vi "p2.vi"() -> ()   [LabVIEW 2021, in "d21.lvlib"]
uses:
  d21.lvlib
  <vilib>/regexp/Match Regular Expression.xnode
  AOC/AOC.lvlib
panel:
  out "Numeric":i64
  out "String":string
  out "Reduced 2":string
  out "Reduced 1":string
  out "side 2":string
  out "side 1":string
  in  "Example":bool
  in  "Example":string="root: pppw + sjmn\ndbpl: 5\ncczh: sllz + lgvd\nzczc: 2\nptdq: humn - dvpt\ndvpt: 3\nlfqf: 4\nhumn: 5\nljgn: 2\nsjmn: drzm * dbpl\nsllz: 4\npppw: cczh / lfqf\nlgvd: ljgn * ptdq\ndrzm: hmdt - zczc\nhmdt: 32"
  in  "variables":string[](array[string])=["fqsj", "fdlt", "zgmz", "rhjl", "snpj", "zvhz", "rldg", "lmll", "stps", "jwbt", "fpmq", "ffpf", "mmmv", "gbzb", "cfjs", "cncf", "mfnp", "jhgz", "mgft", "mrrb", "zllz", "zpdc", "fzvp", "mnmv", "hqfj", "dzjs", "grzz", "zmgd", "mrhm", "pgsb", "hlzf", "qnpr", "fnmj", "nsmc", "dbbn", "gtff", "wrbt", "ztsz", "pqcs", "wlst", "ffls", "ljjm", "vftj", "pggh", "wqpn", "mmmm", "gnfc", "cqnp", "sbvb", "vsmc", "humn", "ggrg", "vccs", "mrgq", "gpgw", "sqrl", "mncr", "rtdb", "lpbw", "ggtj", "drbw", "ztfd", "cbzs", "hhrm", "pnwq", "cwml", "cpbh", "gmmv", "wcrw", "mvgg", "jfcq", "jjpz", "rlqj", "zpgv", "crjg", "bvdp", "hplw", "tfzv", "fnhp", "hzrr", "jstf", "nblh", "lhfc", "wppw", "bdlj", "rpwp", "fbqb", "csrw", "vvwv", "czsz", "pmpb", "fwhb", "bthq", "mzzm", "jngd", "zjqs", "hsbt", "bqtv", "wztp", "hvhf", "fzbh", "bjmt", "bdps", "psqs", "jfpt", "cnpc", "pwdp", "vvmw", "jvzp", "jzsb", "smcz", "hvng", "lftw", "wtvv", "bbbr", "sqsh", "hwbl", "fpnh", "pbrm", "chfb", "zjgv", "rcjj", "whlc", "sgnd", "fhgn", "hzmf", "fztw", "fhpw", "ljvp", "jlqf", "lltd", "vlqj", "tzsm", "mrfb", "ftfr", "lqzb", "pfds", "bbzg", "qgpm", "nlvd", "hgvp", "cnpz", "glsj", "tsrp", "rcdp", "qzml", "mvjr", "gvbp", "dcps", "qjdp", "mqbr", "llbh", "llnq", "zlrl", "ngnd", "vfqn", "grdz", "wtwh", "vhhr", "vtpt", "zjzt", "fdzj", "pgjn", "cbmt", "hpvg", "mmvc", "vhsv", "ffzt", "tcmz", "gctb", "pmrt", "hrvj", "sffd", "mlzs", "qjhc", "qbts", "wpts", "nzlb", "ndpz", "rgqg", "vpdz", "pwbs", "rglt", "dqvg", "pssq", "qvst", "hcjh", "jmzp", "wsnt", "rwgw", "ldzg", "rrtc", "wcpv", "bdlb", "bfcs", "bzzp", "mlrt", "mqzz", "fscv", "qnzd", "nscj", "wrfr", "frbf", "ztfh", "qtmg", "lpft", "vjdn", "rbjt", "ppjv", "cddb", "jqlb", "whvm", "zrwj", "vmzb", "lhwg", "czlv", "vhqj", "svjl", "qrdp", "qnnj", "fbft", "rlbm", "lwlr", "rntv", "cmrf", "tpwz", "mwrq", "lmpr", "zgct", "btcg", "qqwq", "qqdg", "hhqs", "tcgz", "hrsv", "sfjc", "ljhp", "fjzg", "qlfw", "qmjl", "dwms", "szzp", "lvwn", "cmps", "svmc", "fdsq", "ctjd", "gcnn", "pfzr", "jwbq", "mvgf", "wvbq", "ptrm", "hfpm", "tjnh", "vfjf", "pfsj", "vrqf", "ghlb", "pftd", "gsmz", "sjsf", "frtl", "pdhz", "mjbv", "lpwh", "ggzf", "rsbl", "jvct", "wwvz", "ftdw", "stgd", "fdbj", "prgn", "rbgc", "bftf", "lclz", "dspc", "pvzz", "wpjr", "whpl", "mphw", "gnmc", "lnwd", "pcnz", "zznq", "jsml", "sncr", "hhfh", "bbdp", "nqjt", "vsqz", "jdnl", "brhj", "jzmd", "ncdn", "vshf", "psbr", "gznp", "wctd", "qtwp", "pdfn", "shlz", "bqjd", "dssj", "gfwp", "sftl", "lghz", "lwvr", "gjtf", "mmgq", "vqgh", "lmfp", "nbrl", "tlvq", "fjlj", "zrsl", "psgj", "rqmm", "lghr", "lsph", "ztvv", "lwdq", "dmwc", "stwl", "tjsv", "bjbq", "phvh", "gwnp", "lrsm", "qvrn", "rrbs", "pmtv", "rqqf", "twvr", "qqsh", "bwhd", "twvm", "ntnd", "qgrq", "fbjg", "cwbp", "fhtd", "vstv", "hnzz", "fhtv", "hlvn", "fjgb", "vngd", "fccw", "wjpw", "jwzf", "jlvd", "cbcq", "zglp", "nwsv", "hvlr", "rdzq", "bvpn", "hgbm", "qrfg", "gdzt", "tmsq", "pvqg", "vtcj", "bvnt", "pqvc", "zmdn", "qhhl", "sflv", "fsrv", "vvfh", "qbrd", "wgtg", "fthz", "lztw", "hgbc", "fnsr", "lzrf", "qrzs", "vrmn", "cnhc", "whmz", "mcwn", "frrm", "scgw", "jtnp", "dwcc", "nczg", "srbq", "phmc", "wblm", "wchj", "pfsf", "ddwc", "zfff", "vszw", "tnqs", "qmjd", "mpln", "ngpw", "nlnr", "dgsm", "lblg", "grqr", "bfhd", "vwvw", "sgdz", "jsjj", "lzwl", "vpzl", "mqqv", "qtdj", "gjjm", "hpqm", "blqg", "jmrg", "jhsf", "nljz", "djqs", "vhrt", "zqhq", "fqff", "fbcg", "qcwg", "flnv", "qngj", "nzss", "bzhf", "nrhf", "gqhp", "qcfb", "ppnj", "dqbc", "qzsc", "vldv", "bhmq", "rdph", "hhpv", "qtpd", "mrnq", "zfcf", "nvpt", "cdtw", "vthn", "gvmw", "drvd", "nzwf", "rzdl", "cmtj", "jzgc", "trmn", "mdjv", "qfnr", "lmrt", "djzb", "jzjm", "stfl", "jwtf", "hwfw", "gpzf", "pzln", "qgjn", "pvms", "twpc", "cnhl", "fsss", "fvjg", "vnhg", "mmpg", "pmcg", "vmhs", "hfdg", "vjvm", "qsdf", "jfnj", "hmpr", "lndp", "fqph", "lddz", "zjvf", "qfsm", "zgbc", "wdbr", "cfwf", "fmvm", "glvv", "zdlb", "vmjp", "swrj", "pnbt", "tflg", "cvbb", "wrsc", "hvwn", "bmvv", "pbmz", "dspb", "njfr", "vngz", "jqwn", "lhbv", "sjvn", "sccd", "fnhn", "thrp", "djjw", "cpss", "thhv", "sdlc", "dwcs", "zmmg", "jhbp", "zpbt", "cptw", "thqn", "cvjd", "qwfl", "swft", "flcm", "vjvq", "wppp", "gscs", "tjqd", "ssqz", "mlpt", "qshb", "lmhg", "vlqw", "vnjt", "qbtz", "psmz", "bldp", "zlvb", "zldr", "jfpc", "jhfb", "dznt", "qjsm", "wfdf", "ntzq", "dtzp", "jmnq", "pdrl", "rrsr", "ndmt", "vzrw", "cpwh", "mpcq", "dllf", "hhrg", "vqpd", "frtz", "lfrj", "jnwf", "mlmw", "shzm", "ghsv", "wvvd", "bjpf", "dzdz", "bgps", "gstb", "zscg", "wspb", "njmt", "ccfn", "ttsg", "flhq", "clgf", "hpml", "gssz", "bwvv", "nrbl", "wrvb", "cqfp", "sjdv", "hqvl", "mmdv", "wdlq", "fqtj", "hqcw", "pzsw", "bbwd", "cmwv", "zsdb", "zpps", "jhrr", "tcgc", "zgts", "mwwh", "jvbp", "htgt", "sjhh", "tzbj", "rshs", "gjlq", "nbht", "dgrp", "mlwr", "brqf", "vtwf", "crzd", "hwfv", "znrs", "wptb", "qvmv", "fqbs", "mbsr", "qddw", "psmg", "gtlz", "fbnh", "czbt", "mrfd", "gmsl", "nsqh", "trhr", "jmvf", "cbcp", "mssw", "vlth", "rppw", "vcbq", "mbln", "zlth", "vnmj", "gmdz", "tcnw", "hrqc", "jzdw", "lhcc", "wlcf", "vppv", "wpfs", "mzbt", "llwp", "lhlt", "gqth", "jgpl", "gfsn", "hdqf", "mrsr", "gffp", "vnlv", "tmcn", "bgdj", "drzl", "gnzj", "rqbt", "sjpv", "cjtd", "rwth", "jrcm", "gcfh", "lfsw", "gwhg", "msjr", "wcsg", "vtjc", "jrrm", "svdj", "wrnn", "zqns", "fgvl", "jtqc", "hhgq", "ntvw", "pqsm", "gpgv", "fdpb", "srdz", "znqr", "qvtc", "pptp", "czcv", "qszg", "lncj", "rmfw", "ssfw", "rlzq", "dzqz", "pllt", "dcbw", "jnzs", "stjp", "lrwf", "whch", "wpfl", "btqv", "dqvh", "fcgl", "czzd", "gjbv", "prdj", "fgsg", "pptj", "svvz", "zvql", "zwzz", "vrpt", "mwhr", "wcth", "jdvt", "ftcc", "gsdv", "zgnh", "gfrp", "dbhf", "trbc", "ctsb", "wdvw", "lfrq", "wgnp", "mgqq", "lcvr", "lcbg", "qbrw", "rctg", "brpp", "lhwf", "gvht", "njsn", "zbfn", "zpmb", "dqwn", "llfn", "grwz", "dslc", "ndms", "jdzb", "pcbr", "swhv", "qvnm", "dmbb", "vjjj", "fmhp", "jmqw", "bpzj", "dtnn", "ssbz", "jwzp", "shqb", "tpbv", "fgbj", "sqjn", "hbwt", "szlm", "wthv", "bgvh", "thpr", "gddt", "nvwg", "hvgn", "cprg", "gssl", "qlhm", "nbmq", "wrmr", "sdbp", "phtq", "dvhs", "hgsq", "zzzq", "lvmh", "ngwp", "bwgh", "sgnf", "lnrv", "jsvl", "zrqs", "fnzf", "rgnn", "jpsn", "lscv", "cmdh", "tnlt", "dwzf", "mbpn", "hvqw", "qfcb", "flpq", "cchp", "mwmj", "bvfh", "jtth", "tccw", "cjdw", "lngs", "vnhq", "lgnr", "cnlq", "qqpg", "rhwd", "dfwl", "jplw", "ljmz", "rlfr", "nlqz", "gqbc", "dwtr", "zdmt", "pbtd", "zcfd", "gljm", "gcqm", "jqwf", "wjvr", "lnnn", "qwgr", "zlnf", "dbqv", "bclj", "srjd", "bjzg", "plzs", "grhj", "gnjd", "twhl", "nnnd", "thhh", "nhhp", "bfzr", "rcgg", "zrff", "rjmj", "fvss", "fzqd", "tlfp", "mnqb", "ghsl", "bwmb", "jmjw", "msrj", "vwfn", "gpss", "vmgm", "ndhs", "ghlg", "zfrc", "zggn", "bhgs", "rfqr", "blzh", "lvfl", "mpqv", "gqbg", "spbp", "mfcr", "mrdg", "msjl", "twqt", "crnq", "gfjb", "fzjs", "nmlg", "zdgg", "vrzn", "bdhr", "trrb", "smmh", "gpmb", "zlwh", "bhsp", "zplf", "wtzd", "hbqg", "tvvw", "wzvf", "jtss", "vwqm", "jvfm", "ljpj", "shjf", "jfhp", "zdrn", "jgqb", "rqvr", "bhlz", "vlsv", "tjhj", "zcbt", "jbmw", "thjq", "fflh", "vdbm", "ngrc", "ftqq", "lwcv", "czlg", "dlpz", "dmjl", "llfl", "gdmq", "qdwp", "ddzl", "pnhs", "bbfv", "wndp", "bprt", "cvnz", "jfhm", "zflq", "nbgq", "shpf", "bjfv", "dslt", "hchb", "nlgj", "lwpl", "rtcr", "qvhb", "qzhv", "tfqj", "vdmh", "ftdt", "jvrr", "hqth", "vblt", "nprq", "msvm", "dslb", "vpmj", "vdgc", "bfzf", "mhww", "wcjm", "nftf", "wjjn", "qmlr", "tbjd", "sppt", "rdpp", "vbln", "tdfr", "hfrg", "nqzc", "tdwc", "ccwq", "nblt", "rtrm", "gfht", "swgf", "wbwr", "jvsf", "fwzl", "sdsh", "lwlw", "vnts", "qnzq", "qsmb", "qdqj", "nszq", "cpsb", "blpc", "dsql", "vvfm", "ldfr", "hgzd", "ztwf", "ftzl", "wdtb", "mpjc", "tmfg", "mbvw", "fvzt", "rjvd", "msmm", "bpvm", "twjg", "gpcz", "wjfv", "pnft", "swtz", "jljb", "rdms", "qcrj", "tmwh", "rfgp", "ggsw", "tvjg", "qpjg", "pbll", "pbpm", "mdtr", "msqs", "jgsd", "btqc", "rqmd", "sgzm", "srpc", "znqt", "wvgg", "sbrh", "tzsq", "fczq", "fhwj", "bdbl", "pgzr", "fjgt", "jfwh", "srnq", "bvbp", "qlrc", "mlbn", "fdnn", "mmql", "wsql", "tpbz", "ddwg", "lllp", "qmhc", "qhhm", "dmlq", "vlfs", "hrqv", "zjhq", "cbvf", "wgmq", "spgf", "hpcs", "rrnb", "jgrj", "vhcd", "vpfm", "tplj", "gchb", "gzsb", "gqdq", "fpbb", "wbgb", "gpml", "lszf", "rnqw", "dbvt", "tqlv", "rvgs", "qcqd", "drjs", "bfsl", "nldh", "wsbf", "fcfh", "tdjm", "pwwg", "ldgg", "bvjj", "tvfq", "jsgm", "sdmq", "vwcg", "bwfb", "rljt", "tqcw", "ncch", "nttz", "cbjm", "zwdd", "smgm", "tffn", "gnnb", "sdbv", "pjmm", "jpgl", "njjh", "bmcl", "mcmt", "rpgd", "mchw", "vnhp", "snnj", "zmwd", "dbdf", "czzm", "gvtc", "pfdf", "qjmt", "jfsl", "ttmw", "zngb", "wdgr", "dzbl", "sdvq", "llhc", "fmhf", "sndl", "rbjh", "jglv", "nrnc", "fvfv", "hsnb", "lpcp", "rlrj", "qpgd", "bwjj", "fmdv", "prqr", "czjq", "rrfg", "lzcr", "mcdq", "qmlb", "lrbz", "rwjl", "cffn", "bsbs", "fszt", "pmsn", "gjcw", "rscq", "vfdv", "jnzd", "mbjv", "rjtp", "bzpv", "vdtv", "bpcz", "qhpn", "fbqq", "snhj", "nrfq", "cwcg", "hdhq", "tvpj", "gmmw", "mszm", "fhrw", "jvth", "lbzw", "mlwq", "dhln", "mrns", "dzmw", "pdbb", "wwbs", "rnwg", "bfvv", "wmnt", "fllv", "vzhn", "djpp", "rhtm", "tbzz", "rwws", "dpfp", "cshg", "svmf", "cztz", "jhps", "zjwz", "rwgf", "qjcv", "zjth", "zzws", "jmtc", "hhds", "qtnh", "dtfm", "mwsq", "cfmq", "rnqc", "zbmq", "drfs", "dwlp", "pzvs", "tvcv", "jzvj", "hnhv", "slch", "dntj", "wmsr", "snpr", "mjcz", "jjsd", "ndjh", "vnqf", "mvnl", "glln", "crsv", "thss", "mczd", "lcnv", "cghq", "brtm", "jqzz", "mqnc", "lcsg", "fbpf", "flmq", "tldr", "qppc", "mqnr", "bhtb", "dsrc", "sgfw", "tdjh", "frgj", "lcrt", "cjpv", "ssmv", "nzbp", "szjl", "htgj", "hpwh", "gvqg", "nmnr", "zfhv", "pzls", "lmqh", "zcgm", "zhpp", "cbsq", "jgwl", "djwz", "vwbh", "nmcz", "wjzt", "slmh", "jpnz", "sscw", "fqgd", "rlsf", "ggqn", "zbgr", "stds", "pptm", "mfjj", "vsps", "pghb", "vhpn", "mbgv", "srjf", "zprj", "hssb", "vflp", "wqmm", "btmf", "lbzn", "crtg", "hvmn", "qpsl", "rphl", "pbrc", "crps", "ftgq", "brcn", "ttqs", "wrqb", "wggj", "prnn", "mfdd", "tfrz", "llgp", "sqfc", "wssw", "vpvh", "tshp", "qwcf", "jthp", "tqzz", "zvlv", "ntcm", "bwgq", "dfsj", "pldw", "nbsw", "prsz", "mhdv", "zddt", "wjwv", "dljs", "nscr", "vnbh", "scsc", "qhsr", "qsmr", "hghr", "sthl", "jmcr", "rtct", "pldc", "sjzp", "fzhh", "wpjq", "bcdz", "ntvp", "vtbv", "bcdf", "tqsj", "ftvr", "wptm", "qzcj", "wtqq", "rmqh", "vhmc", "znhd", "llnm", "swjq", "jfcn", "fwtt", "jbgz", "lttg", "nghw", "shrv", "cwmh", "hvcm", "tsdl", "lpfz", "sppg", "rgjr", "qjrv", "ftgn", "tscj", "ghmp", "cdrs", "gvrj", "vrnt", "rnnm", "hrcn", "rljv", "pngs", "dndl", "wjvv", "lmvc", "vtgj", "jltn", "ssrb", "rlcj", "frth", "zrdd", "lrpl", "lpsz", "dwsf", "lqrd", "qvdw", "smvb", "pzps", "gpvg", "zqms", "hmdj", "bhzh", "cjdg", "nmtj", "szrj", "tnmt", "phhh", "qsqj", "sgtg", "lvvq", "cmct", "qrgf", "lnzb", "bvjn", "mjzr", "zrbt", "jpwq", "smbv", "vdjf", "zmzd", "vnsf", "glmt", "dgmt", "llhz", "spgn", "dwmn", "fmhb", "pzbj", "lrbs", "bpzr", "bnnt", "pjng", "zgwp", "wgvg", "hjvl", "fvrf", "pqml", "nqft", "vmzt", "mrrw", "fzwq", "mnmr", "lcqq", "lpgv", "srgh", "hmpc", "pbtm", "ncvr", "fclv", "zhtg", "vsnh", "lnsc", "tftq", "mzdw", "pgwr", "qzgr", "czmj", "cscn", "lpnp", "zspd", "vdlr", "nzjt", "ndzb", "thsq", "pdhf", "sgzc", "zmrp", "vphg", "lntt", "cbjl", "vqrf", "sscd", "qcbw", "wfgq", "mgrj", "hqnn", "zdzc", "qght", "cfqb", "lwsn", "hfjh", "vbsr", "vlgr", "rqnt", "pqwg", "sldt", "whcp", "lbvn", "nzlz", "gvhg", "mnjc", "qwrl", "mdlt", "ftth", "chdb", "msdt", "pnlt", "rtpj", "ldnm", "fhhg", "zqfz", "mphc", "pqzg", "dhhr", "hpcj", "wmzc", "srnd", "mrzl", "sdqt", "scvs", "wwhm", "sbcq", "wswp", "swrn", "qffm", "pbpn", "rtvw", "wjbj", "hfgl", "msdc", "lrhg", "hvzv", "jpgf", "djwm", "zfwb", "cwlp", "mhrh", "qmgl", "zzbc", "fsmq", "frrt", "zhrq", "lzhh", "lhfq", "dswf", "jjch", "cmqj", "cwff", "bnrb", "ttvg", "mppd", "nrts", "bblj", "cppb", "gqjt", "phfj", "brwz", "gdzm", "hngs", "frdw", "zvlp", "bltn", "vtsm", "rqtc", "sqbv", "tttp", "thfr", "pmbh", "mqhb", "gwcl", "tqzb", "nwvj", "hszf", "gctg", "sfwc", "ntqz", "nsdj", "zzql", "pvcz", "rrzv", "sdvd", "wrpd", "nmqc", "pgss", "vtbm", "ccrg", "vgtv", "dmjb", "jvcw", "svvl", "dphn", "dwjm", "fzcb", "ddtz", "lffw", "qgzh", "dbrp", "glwr", "hntg", "qhqc", "mhqf", "lzjz", "ptnr", "dzwp", "ftbz", "glvf", "gsgq", "vlms", "gnhg", "rzgj", "cvpc", "sbql", "dqrc", "pwjw", "bddl", "qnsd", "bdzz", "qcmn", "fhlm", "mjnm", "wqmw", "sfzr", "wpwz", "ndvz", "hfhh", "gffm", "pvlf", "wcqv", "chnc", "jzvb", "bngc", "ltqm", "rgqw", "gnbz", "wcrt", "qvfd", "ztsf", "dvlf", "trtj", "dttp", "tvmh", "bqgw", "hbtl", "dcqf", "dffz", "mpmp", "jsvs", "srcm", "rbbr", "dgms", "nvbj", "gstr", "nvfs", "lwbg", "vhlb", "rhqq", "hcvj", "qhdp", "mngp", "gtvr", "msjw", "tfvj", "lmss", "zdtw", "dzmt", "zwdt", "cqsm", "fzdn", "gsnn", "sljs", "tvzt", "qhqj", "fpdb", "fngn", "mprs", "ptlc", "pclv", "zgbp", "vjmb", "zqgm", "tqlt", "bltl", "nnbw", "dghd", "rlhg", "bhzd", "dtwn", "zttv", "bvcg", "jvqh", "zqnf", "rrft", "dlrq", "gfwf", "fhqn", "jfdp", "fwzv", "fgrw", "hwfs", "phrb", "vfwv", "hmpw", "wrts", "jnmh", "qljm", "gqss", "rswn", "sgrr", "ttsz", "mhdr", "bqvv", "zlbw", "qqzp", "gbwj", "hfbj", "rlll", "ctdv", "pdsz", "swwq", "tfgv", "djgl", "qgff", "jmmj", "jswr", "fgld", "jnhf", "jwpf", "mslt", "dgrs", "rbbj", "mccm", "njpj", "wgmf", "lplq", "bcqm", "twdm", "vjcp", "cbqz", "zszs", "rwwp", "lddr", "mgnh", "gfws", "zcbr", "cfwq", "jtfr", "gzmz", "vrzv", "drcm", "nrjz", "sbzv", "tvzz", "jcwg", "rhbg", "pmgb", "vpdq", "lpzw", "dnvb", "ncdr", "lfzc", "qzrn", "vtrz", "cpqm", "srcj", "cgqp", "dtnh", "nbrg", "czts", "jzbc", "dvzm", "qtrf", "nhqw", "hpnh", "vdqq", "crpg", "tjhg", "fvtb", "tfcv", "vtdz", "jgbg", "mmrq", "fsgb", "msnr", "rmfl", "rttb", "wcph", "crcm", "zgfq", "stss", "hrcm", "nsld", "bcwq", "spcp", "rnjn", "cfvb", "bjjn", "gbnz", "vbcn", "cwlv", "rvmp", "pggv", "wscv", "mfsv", "qdwz", "vmlt", "snjj", "ccch", "cslz", "chsf", "qqqc", "jjbj", "gcdw", "qqmb", "szdt", "cscc", "ffzw", "wvhd", "wdrq", "sqmn", "wsdb", "cdjp", "dhfw", "vtvq", "rhnn", "gfds", "mjgq", "fvtd", "zwcf", "thzg", "vlzz", "ptht", "nqhb", "vntl", "sbft", "bmdr", "mvzc", "zngw", "zntj", "znhn", "gddc", "nhrw", "qtfm", "cblf", "bwcj", "dhqh", "qbfz", "svsb", "jhhb", "fcpw", "ddpg", "wshd", "srpm", "ntmq", "gjfb", "ccbw", "hgvb", "hccc", "hgmr", "fvbh", "pdbd", "vssp", "fcmb", "mjgp", "mgtb", "plbl", "hmtj", "htwq", "jgjj", "bgsq", "rqmc", "jvfz", "nzfg", "zsdr", "fgzv", "cgzh", "pqdh", "lrzt", "cmgs", "ttnh", "zsvd", "sjpp", "gvph", "lpzh", "tfbw", "dtjl", "ftjr", "gwbc", "zgvs", "hzfg", "lvpc", "pvtr", "twqf", "mcwz", "mntg", "dtcz", "dqrf", "wblw", "bhwd", "smcf", "vgzv", "qmht", "wsqt", "qmwn", "mdql", "jhzs", "zftn", "cpvd", "gsjf", "gnjw", "lvcp", "bswg", "jpjv", "scsp", "jrnp", "sgcs", "qtmp", "bwgm", "bplm", "pntf", "zghm", "fqlj", "fdqg", "bhgp", "prcd", "ggvq", "tdlf", "cgnr", "ncpn", "lnqc", "wmls", "fpgs", "vnpl", "gqqj", "pdtc", "tqlc", "bfwv", "hpvt", "dqvq", "rfmq", "tvnc", "mftf", "vvpv", "pbfn", "rrsp", "chsg", "pmms", "hbcd", "hvsl", "mcwg", "zzmn", "ppdl", "tbrz", "hczv", "fwtv", "qgjt", "vndc", "tmqf", "ljbn", "lnrr", "dgcq", "lzlb", "tcqz", "rrlf", "dzss", "glbg", "dplg", "nbhf", "jdnj", "pcth", "nqzb", "btzd", "htcn", "tmfm", "lvmv", "lzhg", "zzsp", "rcnl", "bmjr", "hjch", "wjsv", "tpcm", "fgfv", "vmhf", "nrnq", "lvwb", "jnnh", "szrq", "glcz", "jwvb", "ffvr", "dmfd", "nhdf", "bsbt", "dfcv", "nvrc", "hmjc", "mhfc", "hbtt", "jbqj", "zvbs", "jjrp", "bmsj", "mvzv", "tvpc", "gnmd", "srcb", "mwnz", "vjgm", "phwh", "vcdc", "qfsh", "sddl", "grdd", "gdjz", "wqsf", "hgmf", "jmfg", "fdhf", "vgbg", "njwh", "tfpd", "rvzd", "rqqv", "glfc", "fzsj", "lbhs", "bvwz", "svzt", "szhv", "lcvv", "htlz", "fvcs", "rwqr", "msbw", "btmn", "hrqf", "zwpw", "rzgm", "gccl", "ndrd", "swfn", "hjbn", "pjnj", "grws", "mnmn", "mgcj", "scmf", "vsbj", "hnzb", "fdrl", "nmhv", "vdgm", "fzrd", "zhvn", "jpfd", "tvms", "pwdd", "jrbd", "pbht", "ftmm", "cqwl", "tntn", "gtpz", "jqwp", "qfcd", "hfrh", "cftd", "gdzr", "tlsn", "ztfv", "jzhc", "pqlj", "chvn", "npvt", "sddq", "tgsj", "dthz", "tbzf", "vmvd", "qqnc", "wfhj", "vsbc", "dlhh", "grjb", "pjnz", "jcnb", "tvqf", "snbl", "mnhw", "jjsb", "ldrc", "zgnn", "frdh", "pcrq", "rzfv", "pslz", "ltrz", "nljm", "njzd", "pnmp", "czph", "tbpp", "wstn", "dztm", "htcp", "fvsr", "rcln", "njmp", "hfzj", "sgcj", "wrrg", "npdp", "npwg", "pdqh", "jzpn", "wrns", "cjnf", "spgg", "mpqd", "rrvr", "npnc", "crjw", "pgdm", "jpgj", "tpjb", "wptr", "whqn", "llsm", "lwsl", "qtdm", "tfjn", "cczs", "tflv", "jzzt", "ptmq", "hlhj", "pzmc", "rnsc", "gfvb", "tsmw", "tnzf", "vhtm", "bjzj", "rnmz", "vjvl", "hlbl", "trnr", "bttd", "tltr", "tvqz", "blqb", "hczq", "vnml", "tdgw", "wjsw", "prwp", "ppms", "nnvv", "gntm", "tdmc", "gczr", "wbcp", "wzjh", "zhgs", "mpvl", "cgjw", "wsnz", "nhgs", "wzmw", "drfl", "dvgl", "gbrl", "cfpd", "gfjg", "rhfj", "fwjz", "gdgp", "ddqh", "zlnt", "fcvj", "fqpd", "wfrm", "dzqs", "pfps", "jbbv", "jqbd", "pzmm", "jfvl", "mrjc", "pbnl", "wvnm", "mzsr", "htwv", "tsjh", "zdwh", "dnrs", "tnvv", "hfqm", "mgfn", "wlql", "mpmb", "jchf", "nnpf", "nqbm", "srwt", "lwjr", "fwpb", "htzl", "cmjq", "gpsl", "bpms", "mnld", "tfhf", "hdjm", "dngs", "hnnt", "mpqq", "hcbs", "rsrp", "wdjp", "mcgr", "clhs", "zppc", "rgfr", "tmqm", "rcdg", "thfg", "bvqd", "rtqw", "lpdr", "wbwh", "gfjq", "bzdv", "bmrn", "njld", "zjct", "tjgg", "rqht", "jlvb", "pfrc", "psdt", "mpfp", "vlhn", "srjh", "tpch", "tthg", "htmn", "shnl", "pffp", "wbzh", "vjst", "jmdw", "hgqg", "njnh", "ctgb", "fmcp", "rwlt", "wjdf", "mhwj", "bqjr", "pvdd", "vdsp", "bmrv", "mjbr", "wnzb", "rthh", "pdmh", "bhzg", "rflc", "jfrl", "bzsj", "fsjh", "swtj", "zlcq", "fjbs", "rbcm", "cmtg", "zhhh", "rjtr", "fbhc", "bdcr", "mphf", "lbfr", "frlj", "rtwl", "qffw", "pbzz", "lgcs", "hbbw", "bffq", "zwch", "jwpq", "fpnb", "ssdl", "jsfw", "lstd", "mgvw", "vzzc", "glmz", "lrfp", "dgvm", "mqcv", "zbsg", "lzqg", "rtrt", "zvdb", "jgtr", "pbbd", "hjcz", "qhfh", "rvwn", "jtgb", "zshv", "twrj", "qqcd", "rwtd", "dffp", "wqts", "nfgf", "vjjm", "stvh", "mvbm", "rzfm", "ztpv", "prbd", "bnqg", "lfct", "zpdt", "fmfs", "mnfn", "lngc", "ntlc", "rnnc", "rrnj", "mnvt", "rlbq", "gsfw", "zfcl", "cmtw", "fjmv", "lccn", "djft", "mrhg", "fjwp", "zzcr", "qgwj", "bjbj", "sngh", "vrlw", "mzfj", "jzzs", "rhjv", "jhnn", "tpbb", "rjln", "bppv", "jtdz", "hvwz", "lnvl", "gbdb", "sjfl", "fwcs", "mrvp", "zpmt", "wbrj", "wrzn", "cgfp", "pdjq", "cqqr", "lgpm", "cphl", "frms", "sdph", "tqwj", "drgt", "jwjf", "bbcz", "wqnz", "vzlj", "dzhv", "sqmd", "mjbs", "wptl", "mctl", "mwlm", "ghrb", "fnhf", "rfss", "zltc", "bfjw", "swfm", "tzhz", "rhqt", "bqbl", "lqtf", "lhtw", "bscl", "stph", "mlbw", "lgvv", "crcs", "ghnz", "qlzb", "mplm", "rlqr", "cpjm", "rvfq", "bcvw", "jlpl", "pbmf", "bcrh", "vbqc", "fmml", "rrhd", "nsrb", "wznm", "zfdg", "tcvs", "jzpm", "bmnh", "mcnq", "trfm", "mtvl", "llfv", "zdjp", "mmqt", "wpcp", "dsfj", "vcgg", "mbvc", "qtlz", "rwcm", "pzrv", "vgwt", "wzsm", "cjmv", "qbwm", "gsrw", "lbvf", "smwp", "zfdm", "mvdl", "wggs", "qwrb", "qrjj", "gdjw", "vvqb", "wltf", "bjhb", "sjsc", "dsvv", "dnsc", "tjwz", "tptw", "dgzb", "jlwv", "bhbz", "fwhn", "drwv", "rtth", "qbvs", "qmws", "vptz", "wlvv", "qjmb", "qzfc", "gdqd", "jbtg", "blrb", "jzsf", "ltsj", "ctwr", "gnrm", "stlg", "fjrb", "dvjz", "gtss", "wlms", "gnhf", "vlnw", "qqhr", "sjsv", "npsg", "hctf", "pdwf", "hplg", "scbr", "lgpf", "prlb", "ppfb", "gmfl", "bmhv", "nvmj", "jnlb", "stgv", "ctfm", "cdpw", "drjz", "tttd", "pqss", "whlg", "cjqf", "fblp", "ttcw", "vjvp", "jjqm", "grcg", "slqh", "fttn", "wfwb", "tltv", "gjpj", "tpcv", "wbdm", "dhns", "gvhd", "cdpv", "snhs", "gmwp", "pwhs", "chrd", "nrmf", "dnmm", "nnll", "zprm", "pgbt", "sncs", "vrqs", "dvvg", "vnjm", "svhp", "nctt", "rwpb", "llwb", "mpzz", "vfch", "vfhc", "lqwj", "jnsh", "gfzv", "msbs", "rgbw", "smcc", "lvng", "csms", "jlcn", "thbr", "vwqj", "qdhb", "qcqh", "pdgl", "psvq", "vbrz", "dhhz", "mmtv", "twdw", "rqbz", "dbvf", "tcmn", "bhpt", "zgrf", "qgqc", "snlp", "pgpp", "jwhz", "rcqw", "ppvh", "gzws", "wtqv", "dbjp", "lpcj", "pdqg", "qbwz", "hgvz", "vccc", "czsj", "tdfs", "cgcr", "lhvn", "mtwd", "ljwv", "dggh", "lzjb", "gwmn", "zpsl", "fbrs", "fzfl", "hvfn", "tsjl", "vwtf", "zwms", "fmsf", "vrfr", "crvp", "pfmr", "pwgh", "dwdz", "wccw", "tdjf", "qfpc", "zvdc", "nvjh", "cwqd", "nvqn", "dvjw", "pzbs", "thbz", "qnzw", "qrlp", "sclc", "hzlf", "vqpg", "pncq", "cfdc", "qhbw", "vmbf", "vprz", "bzhl", "lmjw", "svqq", "crdp", "glmp", "vfgn", "crtp", "dlrd", "zwrp", "wbvr", "wqhz", "cgtj", "fzqs", "smmg", "bngr", "fzjr", "hscb", "gdvr", "jvzj", "fqwv", "bfbj", "tbgc", "tpfl", "cfsz", "jwmn", "cjvd", "vsch", "mbds", "fqgp", "gmpt", "czhf", "tjvw", "gzzt", "dcgw", "vlqc", "zgnd", "rhlv", "sqnv", "gdlr", "fjnp", "fbzw", "cpds", "pndq", "lhrw", "nnvm", "bqbd", "svtg", "dgng", "bjft", "lntp", "root"]
  in  "Formulas":string[](array[string])=[" 3", " 4", " 2", " 8", " fdlt * fqsj", " 1", " 1", " rhjl + zgmz", " 2", " snpj + zvhz", " 2", " rldg + lmll", " jwbt * stps", " 2", " 3", " 10", " fpmq * ffpf", " 2", " 9", " 19", " 14", " 5", " 5", " cncf + cfjs", " 1", " 3", " 2", " mmmv - gbzb", " 2", " 5", " 3", " zpdc * fzvp", " 18", " 3", " 6", " hqfj + mnmv", " 1", " 13", " 2", " 7", " 17", " 5", " 2", " 15", " 5", " 3", " jhgz * dzjs", " grzz * mgft", " mrrb + zmgd", " mfnp + zllz", " 3951", " 1", " qnpr * pgsb", " 10", " gtff + wrbt", " 2", " ljjm * ztsz", " dbbn + fnmj", " nsmc * hlzf", " vftj * wlst", " pggh * wqpn", " ffls * pqcs", " mrhm * mmmm", " 1", " vsmc * cqnp", " sbvb * gnfc", " humn + vccs", " 4", " mrgq + ggrg", " 2", " gpgw + sqrl", " 2", " 3", " rtdb + mncr", " lpbw + ggtj", " drbw + ztfd", " cbzs + hhrm", " 2", " cwml + pnwq", " 6", " 2", " 4", " 2", " 18", " 3", " 3", " cpbh / jjpz", " gmmv * hplw", " wcrw - tfzv", " fnhp / mvgg", " jfcq + hzrr", " jstf * rlqj", " zpgv + nblh", " lhfc * crjg", " bvdp + wppw", " 19", " 2", " pmpb * rpwp", " fbqb - czsz", " bthq - csrw", " jngd + mzzm", " 5", " zjqs * fwhb", " bdlj * vvwv", " 3", " bjmt * fzbh", " 3", " hvhf + bdps", " hsbt * psqs", " wztp * bqtv", " 2", " 5", " 4", " jfpt * jvzp", " jzsb - cnpc", " vvmw + pwdp", " 5", " 7", " 5", " hvng + smcz", " sqsh + wtvv", " bbbr / lftw", " 13", " 2", " chfb * fpnh", " pbrm * hwbl", " 3", " 5", " 14", " 8", " zjgv + rcjj", " 3", " 10", " sgnd * whlc", " hzmf + fhgn", " 6", " fhpw * fztw", " ljvp * jlqf", " lltd * vlqj", " 6", " 7", " 3", " 4", " 1", " 6", " 13", " 3", " pfds + lqzb", " 2", " qgpm - bbzg", " 5", " nlvd + hgvp", " 11", " 3", " cnpz * ftfr", " glsj * mrfb", " tzsm + tsrp", " 8", " mvjr * qzml", " qjdp / mqbr", " 3", " llbh * llnq", " 5", " ngnd / dcps", " vfqn + zlrl", " grdz * rcdp", " wtwh + gvbp", " 2", " 6", " 1", " 4", " vhhr / zjzt", " 2", " 3", " 11", " 5", " hpvg + cbmt", " fdzj + vhsv", " pgjn + ffzt", " mmvc + vtpt", " 3", " tcmz + gctb", " hrvj * mlzs", " pmrt * sffd", " nzlb + wpts", " rgqg * ndpz", " 18", " qjhc * qbts", " 3", " 3", " vpdz * pwbs", " 3", " 16", " rglt + dqvg", " 3", " 4", " qvst - pssq", " 11", " 2", " hcjh + jmzp", " 2", " wsnt * rwgw", " 4", " 2", " ldzg / rrtc", " 13", " 15", " 8", " bdlb * bzzp", " 2", " mqzz * qnzd", " mlrt * fscv", " 5", " 5", " 1", " frbf * wrfr", " wcpv * ztfh", " nscj * bfcs", " 16", " 3", " 2", " 3", " 6", " qtmg * lpft", " 3", " 2", " 14", " 3", " rbjt + vjdn", " 7", " jqlb + whvm", " cddb * ppjv", " 2", " czlv + lhwg", " zrwj * vmzb", " 3", " 2", " vhqj - svjl", " 13", " 11", " qnnj * qrdp", " 2", " rlbm * fbft", " 13", " rntv + lwlr", " 3", " 13", " 8", " lmpr + mwrq", " tpwz * zgct", " btcg * cmrf", " 7", " qqdg + qqwq", " tcgz * ljhp", " hrsv * hhqs", " qlfw * sfjc", " qmjl + fjzg", " dwms / szzp", " 4", " 2", " lvwn + cmps", " 5", " 5", " 2", " gcnn * pfzr", " 2", " 2", " 5", " jwbq * mvgf", " ptrm / wvbq", " ctjd * fdsq", " vfjf + pfsj", " 5", " 2", " 1", " vrqf * ghlb", " 16", " 3", " 8", " 4", " 13", " 2", " svmc * pftd", " hfpm + tjnh", " 2", " 9", " frtl * sjsf", " pdhz * gsmz", " 4", " 3", " 2", " 2", " wwvz - jvct", " mjbv / lpwh", " fdbj * prgn", " rbgc + bftf", " 6", " dspc * lclz", " 3", " pvzz * wpjr", " 3", " whpl * mphw", " 13", " 4", " 6", " ftdw + gnmc", " stgd + lnwd", " ggzf * rsbl", " 10", " 7", " 8", " 1", " 14", " zznq * pcnz", " jsml + hhfh", " sncr / nqjt", " bbdp * jdnl", " ncdn * jzmd", " brhj * vsqz", " psbr / vshf", " 13", " 2", " 3", " 12", " 14", " pdfn + shlz", " 14", " bqjd + dssj", " sftl + gfwp", " 5", " wctd + lghz", " qtwp * gznp", " vqgh + mmgq", " 2", " nbrl + lmfp", " gjtf * lwvr", " tlvq * fjlj", " lsph * ztvv", " dmwc * lwdq", " tjsv + stwl", " bjbq * phvh", " rqmm + gwnp", " lrsm * lghr", " qvrn * rrbs", " 2", " zrsl + psgj", " 17", " 5", " 6", " 10", " twvr / rqqf", " 3", " pmtv + qqsh", " 5", " 2", " 16", " 13", " ntnd + twvm", " fbjg + qgrq", " 5", " 3", " bwhd + hnzz", " fhtv + cwbp", " vstv + fhtd", " 3", " vngd + hlvn", " jwzf * jlvd", " fccw + wjpw", " cbcq * fjgb", " 2", " 2", " nwsv + zglp", " 2", " 3", " 20", " 2", " rdzq + hgbm", " tmsq / qrfg", " gdzt + pvqg", " hvlr + bvpn", " pqvc + zmdn", " bvnt * vtcj", " qhhl * sflv", " fsrv + vvfh", " 14", " 11", " wgtg * lztw", " qbrd + fthz", " fnsr - lzrf", " 3", " qrzs - hgbc", " 20", " 2", " vrmn - cnhc", " scgw + mcwn", " whmz - frrm", " dwcc + jtnp", " 2", " nczg / srbq", " 7", " phmc + wblm", " pfsf / wchj", " 3", " 2", " 14", " 8", " 2", " 5", " tnqs * vszw", " 8", " 3", " ddwc + zfff", " nlnr * mpln", " dgsm * lblg", " grqr + bfhd", " vwvw * sgdz", " 2", " 4", " 4", " 3", " jsjj / lzwl", " mqqv * vpzl", " 4", " qmjd + ngpw", " 18", " jmrg * blqg", " vhrt * djqs", " 2", " zqhq - hpqm", " fqff + qtdj", " gjjm * fbcg", " nljz * jhsf", " qcwg + flnv", " nzss * bzhf", " 2", " 2", " 5", " 2", " gqhp + nrhf", " 10", " qcfb + qngj", " 2", " 3", " rdph + bhmq", " dqbc * vldv", " hhpv * qzsc", " 2", " 3", " zfcf * ppnj", " qtpd + mrnq", " 4", " 19", " nvpt * cdtw", " gvmw - vthn", " 10", " rzdl / drvd", " cmtj * nzwf", " 4", " 3", " 2", " trmn + jzgc", " 2", " djzb + jzjm", " 18", " stfl * mdjv", " qfnr / lmrt", " 2", " hwfw * jwtf", " 2", " 2", " pvms + gpzf", " 13", " 4", " 4", " 2", " twpc / pzln", " qgjn + cnhl", " 13", " fvjg * fsss", " 2", " 2", " mmpg * pmcg", " hfdg + vmhs", " 3", " vjvm + qsdf", " 3", " 2", " 5", " 5", " 7", " lndp * jfnj", " hmpr / vnhg", " 4", " 13", " wdbr * zgbc", " 4", " qfsm / zjvf", " fqph / lddz", " 2", " 3", " fmvm * cfwf", " 4", " 2", " glvv + zdlb", " swrj + vmjp", " tflg - pnbt", " 1", " 3", " 4", " 2", " 2", " 4", " 5", " wrsc - cvbb", " 2", " pbmz * sjvn", " sccd * vngz", " lhbv * bmvv", " hvwn * dspb", " thrp * fnhn", " jqwn + djjw", " thhv * sdlc", " 4", " njfr * cpss", " zmmg * zpbt", " jhbp + dwcs", " thqn * cptw", " cvjd * qwfl", " flcm - swft", " 6", " 1", " 5", " 10", " 2", " tjqd * wppp", " gscs * vjvq", " 2", " ssqz - mlpt", " 5", " 6", " lmhg + qshb", " vlqw / vnjt", " qbtz + psmz", " 3", " 5", " zlvb * bldp", " jfpc + zldr", " 3", " 11", " 4", " qjsm * dznt", " ntzq + dtzp", " 5", " wfdf * jmnq", " rrsr * pdrl", " vzrw - ndmt", " 2", " 5", " 3", " 2", " mpcq * cpwh", " 2", " dllf * jhfb", " 2", " 2", " lfrj + frtz", " ghsv * wvvd", " 2", " mlmw / bjpf", " jnwf + shzm", " bgps * vqpd", " gstb * dzdz", " hhrg * zscg", " 2", " clgf * ttsg", " 3", " gssz + hpml", " bwvv / wspb", " nrbl * njmt", " flhq + ccfn", " 5", " sjdv / cqfp", " hqvl + mmdv", " wdlq + wrvb", " 5", " 5", " 2", " 2", " 5", " hqcw - pzsw", " bbwd + zsdb", " zpps + cmwv", " fqtj * jhrr", " 2", " 12", " 1", " 4", " 9", " zgts * tcgc", " mwwh * jvbp", " 2", " htgt * sjhh", " 4", " 3", " 11", " 3", " 1", " 14", " 2", " 2", " tzbj - rshs", " 12", " 17", " 2", " 5", " 2", " dgrp + mlwr", " brqf * vtwf", " 2", " gjlq * crzd", " hwfv * nbht", " 4", " qvmv + fqbs", " 1", " 3", " znrs * mbsr", " wptb * qddw", " 19", " 3", " 7", " fbnh + gtlz", " czbt + psmg", " 10", " 3", " 2", " jmvf + mrfd", " cbcp + mssw", " 9", " gmsl * vlth", " nsqh + trhr", " 4", " 3", " zlth + rppw", " vnmj + vcbq", " mbln + gmdz", " 5", " hrqc * tcnw", " 11", " 6", " jzdw * wpfs", " mzbt * llwp", " 3", " 3", " 5", " lhcc + lhlt", " wlcf * gqth", " jgpl / vppv", " 2", " 5", " hdqf + gfsn", " 4", " 5", " 4", " 3", " 3", " 3", " gffp * tmcn", " mrsr + vnlv", " 2", " 12", " drzl + gnzj", " 2", " rqbt + sjpv", " 2", " 3", " 3", " rwth * cjtd", " 2", " 7", " 2", " 2", " 4", " 5", " 11", " 5", " 6", " gcfh - jrcm", " 2", " gwhg - lfsw", " 4", " msjr + bgdj", " 2", " 2", " vtjc + wcsg", " 5", " jrrm * svdj", " 7", " 3", " 1", " 3", " zqns + wrnn", " jtqc * fgvl", " 4", " 2", " hhgq + ntvw", " 1", " gpgv / pqsm", " 1", " 2", " qvtc * znqr", " lncj * pptp", " czcv * rmfw", " qszg + dzqz", " pllt * ssfw", " dcbw + rlzq", " jnzs * stjp", " lrwf + whch", " srdz * fdpb", " 3", " wpfl * btqv", " 5", " fcgl * dqvh", " 3", " 4", " 2", " 3", " 3", " 4", " 1", " 5", " 13", " 2", " 2", " 4", " 2", " 8", " fgsg + pptj", " 4", " 7", " 3", " zwzz * svvz", " zvql + vrpt", " 3", " 2", " 3", " 5", " 5", " wcth * mwhr", " 4", " 2", " 13", " 10", " 19", " ftcc / jdvt", " gsdv + gjbv", " prdj * czzd", " 3", " gfrp + zgnh", " lfrq + ctsb", " mgqq + lcvr", " 2", " wdvw + wgnp", " brpp + trbc", " 2", " lcbg + qbrw", " dbhf + lhwf", " zbfn * gvht", " rctg * njsn", " 2", " grwz * llfn", " ndms + dslc", " 17", " 3", " jdzb * pcbr", " 4", " qvnm * swhv", " vjjj - dmbb", " 4", " 6", " fmhp * jmqw", " 2", " bpzj * dtnn", " 4", " ssbz * jwzp", " shqb * tpbv", " 4", " 7", " 16", " 6", " 7", " 5", " 3", " sqjn * fgbj", " 11", " hbwt + szlm", " 2", " 2", " 5", " 2", " 5", " wthv * bgvh", " 2", " thpr + gddt", " 3", " 11", " 10", " 2", " 5", " 2", " 2", " hvgn + nvwg", " 2", " 3", " 4", " 9", " 4", " dqwn * zpmb", " 2", " 1", " gssl + cprg", " 7", " 12", " 2", " 7", " sdbp + wrmr", " dvhs * phtq", " 20", " qlhm * nbmq", " zzzq * hgsq", " 5", " ngwp * lvmh", " sgnf + bwgh", " 5", " 5", " 3", " 6", " 7", " jsvl * lnrv", " 3", " 1", " 2", " 7", " fnzf + zrqs", " rgnn + jpsn", " 6", " cmdh + lscv", " 3", " tnlt * dwzf", " 7", " 20", " 19", " hvqw / mbpn", " 8", " 10", " 1", " 2", " 10", " flpq - qfcb", " 2", " 5", " mwmj / cchp", " 4", " 5", " 7", " bvfh + jtth", " 4", " 3", " 3", " 8", " 3", " tccw + cjdw", " 3", " 2", " vnhq + lngs", " cnlq + lgnr", " 3", " 5", " 2", " 2", " qqpg + rhwd", " jplw * dfwl", " 1", " rlfr * ljmz", " nlqz + gqbc", " zdmt * dwtr", " zcfd * pbtd", " 2", " 4", " 3", " 3", " 10", " lnnn * wjvr", " qwgr * gljm", " gcqm * jqwf", " 8", " zlnf / dbqv", " bclj + srjd", " 2", " 3", " 14", " 2", " plzs + bjzg", " 7", " 2", " 12", " 3", " grhj + nnnd", " thhh * gnjd", " 3", " 12", " twhl + nhhp", " 16", " 1", " bfzr * rcgg", " rjmj + zrff", " 2", " mnqb * bwmb", " tlfp - ghsl", " msrj * jmjw", " vwfn * gpss", " 2", " fvss + fzqd", " bhgs * zggn", " rfqr * lvfl", " mpqv + blzh", " 2", " 9", " gqbg * mfcr", " mrdg + spbp", " 8", " 4", " twqt + msjl", " 5", " 3", " 19", " 2", " gfjb * crnq", " fzjs + zdgg", " nmlg * vrzn", " 7", " 13", " 6", " zfrc + ndhs", " ghlg * vmgm", " 2", " bdhr + trrb", " 14", " 2", " gpmb + bhsp", " zlwh + smmh", " wtzd * tvvw", " hbqg * zplf", " wzvf * jtss", " 5", " 2", " 4", " jvfm * vwqm", " 2", " 7", " 2", " 3", " zdrn + jfhp", " vlsv / rqvr", " jgqb * bhlz", " 6", " zcbt + tjhj", " vdbm * thjq", " jbmw * fflh", " ljpj * shjf", " 2", " 11", " ngrc * ftqq", " 5", " czlg * lwcv", " dmjl * gdmq", " dlpz + llfl", " 20", " ddzl + qdwp", " 7", " 2", " 4", " pnhs + bbfv", " 3", " 2", " 3", " 3", " 9", " 8", " 2", " bprt - wndp", " 2", " cvnz * jfhm", " zflq * nbgq", " 10", " 3", " 5", " shpf * bjfv", " dslt + hchb", " 1", " nlgj * lwpl", " 2", " qvhb * rtcr", " 10", " 1", " 3", " 3", " 3", " tfqj - qzhv", " vdmh / ftdt", " 2", " 3", " 17", " nprq + vblt", " dslb * msvm", " 2", " jvrr + hqth", " 7", " 3", " 3", " 8", " wcjm * mhww", " wjjn + nftf", " rdpp * sppt", " vbln * tdfr", " qmlr * tbjd", " 2", " 13", " 18", " 2", " nblt * rtrm", " nqzc / hfrg", " ccwq + tdwc", " vpmj * gfht", " vdgc - bfzf", " 2", " 7", " 8", " 4", " wbwr + swgf", " 2", " 2", " jvsf * fwzl", " sdsh * lwlw", " 3", " 11", " 2", " 2", " vnts + qnzq", " qsmb + qdqj", " cpsb + nszq", " blpc + dsql", " ldfr * vvfm", " 4", " 17", " 2", " 3", " 3", " 14", " hgzd * ztwf", " 12", " wdtb * ftzl", " 8", " mpjc * tmfg", " fvzt * mbvw", " msmm + rjvd", " 3", " 3", " 2", " bpvm * twjg", " 3", " gpcz + wjfv", " 5", " pnft + swtz", " 5", " 2", " 5", " 18", " 1", " rdms + jljb", " 2", " 8", " qcrj + tmwh", " rfgp * ggsw", " 4", " 2", " 3", " tvjg + qpjg", " 5", " pbpm * pbll", " mdtr * msqs", " btqc + jgsd", " 4", " 3", " 3", " 3", " rqmd + sgzm", " znqt / srpc", " 5", " wvgg + sbrh", " 10", " tzsq * fczq", " 1", " bdbl + fhwj", " fjgt + pgzr", " 2", " srnq / jfwh", " 5", " 3", " 5", " 13", " 4", " 18", " 5", " 5", " qlrc + bvbp", " 3", " 4", " 3", " 5", " 19", " mlbn * fdnn", " 5", " 5", " 3", " mmql * wsql", " 4", " 2", " 5", " 3", " 5", " 3", " 7", " tpbz / ddwg", " qhhm * qmhc", " 5", " 4", " dmlq / vlfs", " 4", " hrqv / lllp", " 2", " 2", " wgmq + spgf", " 2", " zjhq * cbvf", " vpfm + vhcd", " jgrj * tplj", " 2", " gzsb + gchb", " 17", " 3", " wbgb + fpbb", " gpml * gqdq", " rrnb - hpcs", " 3", " 5", " rnqw + lszf", " qcqd * rvgs", " 5", " drjs / bfsl", " 14", " tqlv * dbvt", " 2", " 3", " 2", " wsbf / nldh", " fcfh + tdjm", " 2", " 19", " 2", " pwwg * bvjj", " ldgg * tvfq", " 3", " sdmq + jsgm", " 9", " 3", " bwfb / vwcg", " 3", " tqcw - rljt", " 16", " cbjm * zwdd", " smgm * tffn", " gnnb + sdbv", " jpgl + pjmm", " bmcl * njjh", " 2", " 2", " mcmt * rpgd", " 5", " 2", " mchw * ncch", " nttz * vnhp", " zmwd * snnj", " 5", " 5", " 5", " 2", " 4", " czzm + dbdf", " 2", " 20", " 2", " 4", " 3", " 5", " 2", " 3", " pfdf + gvtc", " jfsl + qjmt", " 2", " ttmw / wdgr", " dzbl * zngb", " 15", " 4", " sdvq / fmhf", " llhc + sndl", " 2", " 5", " 4", " 2", " 2", " rbjh * jglv", " nrnc * fvfv", " 1", " hsnb - lpcp", " 3", " 3", " 3", " 5", " 2", " rlrj * qpgd", " 3", " prqr * fmdv", " bwjj * czjq", " 3", " 4", " 8", " lzcr * rrfg", " 2", " 19", " mcdq - qmlb", " 3", " rwjl * cffn", " bsbs + lrbz", " 9", " pmsn * fszt", " 2", " 19", " rscq * vfdv", " jnzd + gjcw", " 2", " 6", " 2", " 5", " mbjv * rjtp", " 3", " 3", " 7", " 2", " 3", " bpcz * vdtv", " qhpn * bzpv", " fbqq * snhj", " 3", " cwcg * hdhq", " tvpj * nrfq", " 18", " 4", " mszm + gmmw", " 4", " 3", " 3", " 3", " 2", " 2", " 6", " 4", " jvth * mlwq", " fhrw * lbzw", " mrns * dhln", " 3", " 2", " bfvv * wwbs", " rnwg * wmnt", " fllv - pdbb", " vzhn * dzmw", " 2", " djpp * rhtm", " 7", " 4", " 2", " 2", " rwws + tbzz", " 2", " 3", " 16", " 3", " 3", " 3", " 3", " cshg - dpfp", " svmf * cztz", " jhps * zjwz", " qjcv + rwgf", " 2", " 13", " 3", " zzws * zjth", " 5", " 9", " jmtc * hhds", " cfmq + mwsq", " 4", " 11", " 20", " drfs * zbmq", " 15", " pzvs * dwlp", " 17", " tvcv * jzvj", " hnhv * slch", " 10", " 12", " 15", " wmsr - dntj", " snpr * mjcz", " 5", " 2", " jjsd * ndjh", " 13", " 2", " mvnl * vnqf", " 14", " 2", " 11", " thss + crsv", " 4", " mczd - lcnv", " 3", " 3", " 2", " 5", " 2", " cghq + brtm", " 4", " 3", " 5", " 2", " glln * jqzz", " mqnc * lcsg", " flmq + fbpf", " 2", " 3", " 8", " tldr + qppc", " 5", " 5", " 2", " mqnr / bhtb", " sgfw * dsrc", " frgj + tdjh", " lcrt * cjpv", " 2", " ssmv / nzbp", " 3", " szjl + htgj", " 2", " hpwh * gvqg", " nmnr * zfhv", " 2", " lmqh * pzls", " zcgm + zhpp", " cbsq * jgwl", " vwbh * djwz", " nmcz * wjzt", " jpnz * slmh", " 5", " 2", " sscw + fqgd", " 2", " ggqn + rlsf", " 2", " 5", " 10", " stds * zbgr", " 2", " mfjj * pptm", " 3", " 3", " 4", " 2", " 10", " vsps + pghb", " 2", " mbgv * vhpn", " zprj + srjf", " 8", " hssb + vflp", " 1", " 7", " btmf / wqmm", " 12", " 5", " 2", " crtg * lbzn", " hvmn + qpsl", " rphl + pbrc", " 1", " crps * ftgq", " ttqs * brcn", " wggj * wrqb", " mfdd + prnn", " 2", " llgp * tfrz", " sqfc - wssw", " vpvh * tshp", " 2", " 2", " jthp * qwcf", " 17", " 1", " 10", " 12", " 13", " zvlv * tqzz", " ntcm * bwgq", " dfsj + pldw", " 2", " 2", " nbsw * prsz", " zddt * mhdv", " 2", " 3", " 4", " dljs * wjwv", " 2", " nscr * vnbh", " 1", " 5", " scsc * rnqc", " qsmr * qhsr", " dtfm + qtnh", " 4", " 3", " 19", " 2", " hghr - sthl", " 2", " 16", " jmcr * rtct", " 10", " sjzp - fzhh", " 2", " pldc * wpjq", " bcdz / ntvp", " 13", " 17", " bcdf + vtbv", " 5", " tqsj * ftvr", " 6", " 2", " 4", " wtqq * rmqh", " 14", " 2", " qzcj * wptm", " 8", " 3", " 2", " jfcn * fwtt", " 3", " 2", " lttg + jbgz", " 2", " 4", " 13", " swjq * llnm", " 2", " 5", " vhmc - znhd", " cwmh * hvcm", " 2", " 3", " nghw * shrv", " sppg + rgjr", " ftgn + qjrv", " ghmp + tscj", " 4", " 11", " gvrj * cdrs", " rnnm + vrnt", " hrcn + rljv", " 4", " pngs + dndl", " lmvc - wjvv", " 5", " vtgj * jltn", " 19", " ssrb * rlcj", " 2", " frth * zrdd", " lpsz + lrpl", " smvb * qvdw", " pzps * gpvg", " hmdj * zqms", " 4", " 3", " cjdg + bhzh", " nmtj * szrj", " tnmt + phhh", " dwsf + lqrd", " sgtg * qsqj", " 2", " 5", " lvvq + cmct", " 2", " qrgf * lnzb", " 11", " 5", " 8", " mjzr * bvjn", " tsdl * lpfz", " 13", " 3", " 2", " 3", " jpwq * zrbt", " 3", " vnsf + zmzd", " dgmt * glmt", " 11", " llhz * spgn", " 2", " 13", " 11", " 12", " 5", " fmhb * dwmn", " pzbj + lrbs", " bnnt * bpzr", " zgwp + pjng", " 5", " 7", " wgvg + hjvl", " pqml * fvrf", " 1", " nqft * vmzt", " fzwq + mrrw", " 2", " 4", " lcqq * mnmr", " 5", " srgh - lpgv", " 4", " pbtm + hmpc", " 3", " 5", " 3", " 7", " 8", " 13", " smbv * vdjf", " 2", " 2", " 3", " 12", " qzgr / czmj", " cscn - lpnp", " vdlr + zspd", " 2", " 11", " 8", " ncvr * fclv", " 1", " zhtg * lnsc", " tftq + mzdw", " 3", " nzjt + ndzb", " 1", " 13", " 3", " pdhf * thsq", " 4", " 7", " 5", " zmrp * sgzc", " lntt - cbjl", " sscd + vqrf", " qcbw * wfgq", " 8", " mgrj + vphg", " 4", " 3", " hqnn * zdzc", " 5", " lwsn + cfqb", " 9", " 4", " hfjh + vbsr", " 1", " vlgr + rqnt", " pqwg + sldt", " whcp * lbvn", " gvhg / nzlz", " 16", " 2", " 4", " qwrl * mnjc", " mdlt * qght", " 1", " chdb - vsnh", " pgwr + ftth", " rtpj + pnlt", " 19", " msdt + ldnm", " 5", " 3", " 11", " 18", " 12", " zqfz + fhhg", " 6", " 7", " 1", " 4", " mphc * wmzc", " dhhr * srnd", " hpcj + pqzg", " scvs - sdqt", " 2", " 13", " 1", " 7", " sbcq + swrn", " qffm + wwhm", " pbpn - wswp", " mrzl * rtvw", " 5", " 3", " 6", " 6", " zfwb + djwm", " 12", " msdc * lrhg", " 1", " jpgf * hvzv", " 3", " wjbj * hfgl", " mhrh + cwlp", " 3", " qmgl + zzbc", " lhfq * zhrq", " 4", " 3", " bnrb * ttvg", " 3", " dswf * jjch", " 11", " 2", " zvlp - frdw", " 14", " frrt * fsmq", " lzhh * cmqj", " 17", " 13", " 2", " 6", " 11", " tttp + sqbv", " pmbh / thfr", " 2", " 9", " 2", " gwcl + mqhb", " sfwc + gctg", " 2", " pvcz + zzql", " nsdj * ntqz", " 3", " vtbm + pgss", " vgtv * ccrg", " 2", " dmjb + jvcw", " 3", " rrzv * sdvd", " 2", " hszf + nwvj", " wrpd * tqzb", " 17", " 4", " svvl * nmqc", " dwjm / dphn", " qhqc + mhqf", " ptnr + lzjz", " dzwp * ftbz", " 2", " vlms * gnhg", " sbql * glvf", " gsgq * rzgj", " pwjw * cvpc", " dqrc * bddl", " qnsd + bdzz", " 5", " qcmn + fhlm", " 2", " mjnm * sfzr", " wpwz + wqmw", " 3", " 3", " 3", " 3", " 3", " 5", " ndvz * hfhh", " 1", " 10", " gffm * pvlf", " 9", " 2", " nrts - mppd", " bblj * cwff", " gqjt - cppb", " hngs + gdzm", " bltn + vtsm", " phfj + fzcb", " brwz * rqtc", " 3", " ddtz + lffw", " qgzh * dbrp", " 4", " trtj + dvlf", " dttp * tvmh", " 2", " bqgw + hbtl", " 1", " qvfd + ztsf", " 2", " 2", " 4", " wcqv + glwr", " chnc * hntg", " jzvb * ltqm", " rgqw * gnbz", " 5", " 4", " dcqf + wcrt", " 12", " mpmp + dffz", " gstr * nvbj", " jsvs * srcm", " 4", " rbbr + dgms", " vhlb * rhqq", " lwbg * nvfs", " 18", " 5", " 2", " msjw * gtvr", " hcvj + mngp", " tfvj * qhdp", " zdtw * lmss", " dzmt + zwdt", " 11", " 1", " tvzt + fzdn", " 3", " fpdb + fngn", " 4", " mprs + sljs", " 3", " 3", " vjmb / zgbp", " 3", " pclv * ptlc", " qhqj + gsnn", " cqsm * zqgm", " bngc + tqlt", " 2", " bltl * nnbw", " 7", " dghd + rlhg", " dtwn * bhzd", " 4", " 5", " 17", " zttv * bvcg", " zqnf * jvqh", " 3", " dlrq + rrft", " gfwf + fhqn", " jfdp * fwzv", " fgrw + hwfs", " 3", " 5", " qljm / jnmh", " rswn * gqss", " phrb * vfwv", " wrts + sgrr", " 2", " 3", " 2", " ttsz * mhdr", " 19", " 4", " hmpw * bqvv", " 3", " 6", " 1", " qqzp - zlbw", " 1", " 7", " 3", " rlll + hfbj", " ctdv + pdsz", " swwq + gbwj", " 8", " qgff + tfgv", " 3", " jmmj / djgl", " 3", " jswr + jwpf", " tvzz * sbzv", " 7", " rhbg + jcwg", " 4", " fgld * jnhf", " 4", " 20", " lddr - rwwp", " gfws - mgnh", " 2", " dgrs * mccm", " zcbr * cfwq", " gzmz * jtfr", " vrzv * drcm", " nrjz * pmgb", " 8", " vpdq / lpzw", " 2", " 3", " 2", " dnvb - ncdr", " qzrn * lfzc", " vtrz + cpqm", " 7", " cgqp + dtnh", " srcj * nbrg", " dvzm + jzbc", " qtrf + nhqw", " hpnh * vdqq", " 14", " tjhg * crpg", " 2", " 5", " tfcv + fvtb", " 2", " vtdz * jgbg", " mmrq * fsgb", " 9", " 3", " msnr * rmfl", " rttb + czts", " 17", " zgfq + stss", " wcph + crcm", " 4", " 3", " 5", " 5", " 3", " rbbj * mslt", " lplq + bcqm", " 4", " twdm * vjcp", " 3", " 7", " nsld - hrcm", " njpj * bcwq", " wgmf - spcp", " cfvb * rnjn", " 2", " bjjn + gbnz", " 4", " vbcn + cwlv", " pggv * rvmp", " zszs * cbqz", " 7", " qdwz * vmlt", " 5", " 19", " 3", " 3", " 3", " qqqc * gcdw", " jjbj + qqmb", " 3", " 7", " szdt * ffzw", " wvhd * cscc", " sqmn + wdrq", " 3", " wscv + mfsv", " ccch + snjj", " 4", " cdjp + vtvq", " 4", " wsdb * dhfw", " gfds - rhnn", " 2", " 1", " 11", " 5", " mjgq * fvtd", " vlzz * zwcf", " thzg + ptht", " sbft + nqhb", " bmdr + vntl", " 7", " 6", " 2", " 3", " 5", " 1", " znhn * cblf", " mvzc + nhrw", " qtfm * zntj", " gddc * zngw", " bwcj * qbfz", " dhqh + svsb", " 10", " fcpw + jhhb", " ddpg / wshd", " 9", " 2", " srpm + ntmq", " gjfb + cslz", " hccc * ccbw", " hgmr + hgvb", " fvbh * pdbd", " fcmb / vssp", " mjgp + mgtb", " 2", " chsf + plbl", " 2", " 2", " 5", " 5", " hmtj - htwq", " jvfz * rqmc", " nzfg * fgzv", " zsdr + cgzh", " 10", " lrzt * bgsq", " jgjj + pqdh", " 7", " 3", " 2", " cmgs + ttnh", " zsvd - sjpp", " 5", " 13", " mcwz / mntg", " dtcz + dqrf", " 8", " zgvs - gwbc", " 18", " 7", " gvph * lpzh", " 4", " 2", " 2", " ftjr * hzfg", " dtjl * tfbw", " 2", " 5", " 2", " 2", " zftn + jhzs", " cpvd * gsjf", " 4", " gnjw / lvcp", " pvtr * twqf", " lvpc - wblw", " 8", " 4", " bswg * jpjv", " 2", " jrnp + scsp", " sgcs * qtmp", " bwgm + bplm", " 18", " 6", " 15", " pntf - zghm", " 7", " fqlj * fdqg", " bhgp * prcd", " ggvq * tdlf", " ncpn * cgnr", " lnqc * wmls", " vnpl * fpgs", " 12", " pdtc + gqqj", " bfwv * tqlc", " hpvt + dqvq", " 13", " 2", " rfmq * tvnc", " 2", " bhwd * smcf", " rrsp * pbfn", " pmms + chsg", " 2", " hvsl - hbcd", " 20", " 3", " 4", " vvpv + mftf", " mcwg + zzmn", " ppdl - qmwn", " 3", " fwtv * hczv", " 4", " 3", " vndc + qgjt", " mdql / tbrz", " vgzv + tmqf", " qmht * wsqt", " lnrr - ljbn", " lzlb * tcqz", " 10", " glbg + dplg", " 5", " 5", " jdnj * nbhf", " 2", " dzss * rrlf", " 2", " pcth + nqzb", " 5", " 7", " 2", " btzd * htcn", " 3", " 2", " 18", " rcnl * lzhg", " zzsp + bmjr", " wjsv * hjch", " 2", " vmhf + tpcm", " nrnq - fgfv", " 3", " jnnh + lvwb", " 2", " szrq + glcz", " 13", " ffvr + jwvb", " 1", " dmfd * nhdf", " bsbt + dfcv", " 1", " nvrc + mhfc", " hbtt * hmjc", " zvbs + jbqj", " 3", " jjrp + mvzv", " bmsj + tvpc", " srcb * gnmd", " 3", " 9", " 3", " 20", " 3", " tmfm * mwnz", " 2", " 6", " 2", " vjgm + phwh", " 2", " qfsh + vcdc", " sddl * grdd", " 2", " 14", " 5", " 2", " 4", " wqsf * gdjz", " 2", " dgcq + lvmv", " 3", " 8", " 3", " fdhf * jmfg", " tfpd * njwh", " rvzd * rqqv", " fzsj + glfc", " vgbg / hgmf", " 12", " 6", " 2", " 5", " lbhs * bvwz", " 10", " 2", " 3", " svzt * szhv", " 7", " rwqr + fvcs", " gdzr * hfrh", " qfcd + cftd", " pqlj * ztfv", " tlsn * jzhc", " fdrl / vsbj", " hnzb / scmf", " chvn * jqwp", " sddq / gtpz", " vdgm / nmhv", " 5", " msbw + btmn", " 4", " 2", " zwpw + hrqf", " rzgm + ndrd", " swfn * fzrd", " tvms * jpfd", " npvt / tgsj", " pwdd * tntn", " 6", " tbzf * dthz", " 2", " vmvd + vsbc", " dlhh * qqnc", " pjnz + jcnb", " grjb * tvqf", " htlz * lcvv", " 2", " hjbn * gccl", " grws + pjnj", " wfhj + zhvn", " frdh / pcrq", " rzfv + pslz", " mnhw + snbl", " zgnn * jjsb", " cqwl * pbht", " jrbd * ftmm", " mgcj * ltrz", " czph - tbpp", " 4", " rcln * fvsr", " dztm * htcp", " wstn * njmp", " hfzj * sgcj", " npdp * wrrg", " npwg * pdqh", " nljm * njzd", " 5", " mpqd * spgg", " npnc * rrvr", " pgdm - crjw", " 4", " 10", " tpjb * jpgj", " 2", " wptr * whqn", " 3", " llsm * lwsl", " tfjn + qtdm", " tflv + cczs", " ptmq + jzzt", " pzmc * hlhj", " gfvb + rnsc", " tsmw * tnzf", " 2", " 5", " bjzj * vhtm", " rnmz - vjvl", " ldrc * mnmn", " cjnf / jzpn", " pnmp + wrns", " 1", " bttd * trnr", " 3", " 10", " 4", " tvqz / tltr", " 4", " 3", " 5", " 8", " vnml / blqb", " hczq * tdgw", " 11", " wjsw * prwp", " 4", " nnvv + ppms", " gntm + gczr", " hlbl / tdmc", " 1", " 12", " 16", " 15", " 2", " 7", " wbcp + wzjh", " 2", " zhgs * mpvl", " 5", " 5", " wzmw + nhgs", " 1", " drfl * dvgl", " cfpd * gbrl", " 1", " 9", " 1", " 6", " cgjw + wsnz", " fqpd + wfrm", " mrjc * pbnl", " jbbv * jqbd", " pfps + dzqs", " tsjh + htwv", " zdwh + dnrs", " jfvl + pzmm", " tnvv + hfqm", " 2", " mgfn + wlql", " 3", " rhfj * zlnt", " jchf * mpmb", " nnpf - nqbm", " srwt * lwjr", " 5", " 20", " fcvj * fwjz", " wvnm * gdgp", " ddqh * gfjg", " 16", " 1", " 5", " 20", " 5", " 8", " 5", " mnld * tfhf", " 3", " fwpb - mzsr", " cmjq / htzl", " 20", " gpsl * bpms", " rsrp - wdjp", " hdjm * dngs", " rgfr + zppc", " rcdg - tmqm", " 2", " 2", " rtqw + lpdr", " gfjq * wbwh", " bzdv * bmrn", " zjct / njld", " tjgg * rqht", " jlvb * pfrc", " mpfp + psdt", " 1", " mpqq + hnnt", " clhs + mcgr", " 3", " vlhn + srjh", " 2", " 3", " 11", " 3", " 6", " shnl * htmn", " 6", " hcbs * bvqd", " thfg + pffp", " 3", " hgqg + jmdw", " wbzh + vjst", " 5", " ctgb - njnh", " 5", " 7", " 2", " 2", " 3", " 9", " 2", " rwlt + fmcp", " wjdf + mhwj", " 4", " 2", " pvdd + bqjr", " 4", " 2", " bmrv - vdsp", " wnzb * mjbr", " 4", " pdmh * rthh", " rflc - bhzg", " 2", " 5", " bzsj + jfrl", " 9", " fsjh + swtj", " 3", " 2", " 17", " zlcq * fjbs", " 5", " 2", " 2", " 4", " tthg + tpch", " 2", " cmtg * rbcm", " zhhh * rjtr", " bdcr * fbhc", " mphf + lbfr", " 14", " 11", " 2", " qffw + pbzz", " hbbw - lgcs", " 13", " frlj + rtwl", " fpnb + bffq", " zwch + jwpq", " jsfw + ssdl", " rtrt * zbsg", " zvdb + lzqg", " qqcd - rvwn", " 18", " mqcv + mgvw", " glmz / vzzc", " fmfs / zpdt", " 3", " 2", " lngc + dffp", " ntlc * prbd", " rnnc * bnqg", " mnvt * rrnj", " 4", " twrj * rwtd", " 2", " lstd * lrfp", " hjcz + jgtr", " pbbd + dgvm", " 2", " 3", " 2", " stvh + fjwp", " rzfm * zzcr", " qgwj + mnfn", " bjbj + rlbq", " 11", " 2", " jzzs * mzfj", " qhfh * jtgb", " wqts + zshv", " vjjm + nfgf", " 20", " ztpv + mvbm", " gsfw * lfct", " 10", " mrhg * hvwz", " lnvl * gbdb", " 2", " zfcl * sjfl", " fwcs * cmtw", " fjmv / mrvp", " zpmt + lccn", " wrzn * wbrj", " 2", " pdjq * cgfp", " lgpm + cqqr", " vrlw - sngh", " 4", " 3", " jhnn * rhjv", " frms + cphl", " tpbb * sdph", " drgt + tqwj", " jwjf + bbcz", " vzlj * wqnz", " 15", " sqmd * dzhv", " 2", " wptl + mjbs", " 19", " rjln * mctl", " ghrb * mwlm", " 6", " 16", " fnhf * bppv", " jtdz * djft", " 4", " zltc * rfss", " 4", " 3", " 8", " 4", " 13", " 4", " lqtf * lhtw", " 8", " bscl + bfjw", " swfm - tzhz", " bqbl * mlbw", " rhqt * stph", " qlzb + mplm", " lgvv + crcs", " vbqc + nsrb", " fmml + rrhd", " zdjp * bcrh", " mmqt + wpcp", " cpjm + ghnz", " dsfj * zfdg", " rvfq * rlqr", " 3", " bcvw + jlpl", " pbmf + wznm", " jzpm * tcvs", " mtvl * llfv", " 1", " bmnh + mcnq", " trfm + vcgg", " 13", " lbvf - mbvc", " smwp * zfdm", " 3", " 5", " 4", " rwcm * qwrb", " pzrv - qrjj", " wggs + mvdl", " vvqb * vgwt", " wltf * wzsm", " 4", " 7", " bjhb * cjmv", " qbwm * sjsc", " tjwz + dsvv", " dnsc + tptw", " 6", " dgzb / jlwv", " bhbz * drwv", " rtth + fwhn", " 5", " qbvs * qmws", " 7", " 3", " wlvv + vptz", " qjmb + qzfc", " qtlz - gsrw", " 5", " 11", " jbtg + gdjw", " gdqd + blrb", " 2", " dvjz * gtss", " ctwr + gnrm", " 3", " wlms + fjrb", " stlg * gnhf", " vlnw + qqhr", " sjsv + npsg", " 1", " 4", " ltsj / jzsf", " hplg + scbr", " 3", " 7", " ppfb * lgpf", " bmhv + prlb", " 2", " nvmj * jnlb", " 4", " 3", " jjqm + stgv", " grcg - ctfm", " pqss * slqh", " ttcw + fblp", " cdpw + drjz", " tltv + tttd", " wfwb * whlg", " gjpj + tpcv", " dhns + wbdm", " hctf * gmfl", " snhs * gmwp", " pwhs + chrd", " dnmm * nrmf", " 2", " zprm * nnll", " 5", " 6", " 1", " 5", " 2", " vjvp + cjqf", " sncs * fttn", " pgbt * vrqs", " 3", " dvvg * vnjm", " 7", " nctt + svhp", " pdwf * rwpb", " gvhd - cdpv", " 5", " vfch * gfzv", " vfhc - msbs", " jnsh / rgbw", " llwb * smcc", " lqwj + mpzz", " lvng * csms", " dhhz * mmtv", " jlcn + pdgl", " tcmn + dbvf", " bhpt * zgrf", " 2", " pgpp + jwhz", " 2", " qdhb + vbrz", " qcqh * rcqw", " gzws * ppvh", " twdw / psvq", " dbjp + wtqv", " 2", " rqbz * lpcj", " pdqg * qbwz", " vccc + hgvz", " 3", " czsj * tdfs", " 2", " cgcr * lhvn", " 7", " 2", " qgqc * mtwd", " snlp + ljwv", " vwqj + thbr", " zpsl + lzjb", " fbrs + fzfl", " 5", " dggh * gwmn", " hvfn + tsjl", " tdjf * wccw", " qfpc * zvdc", " 2", " 2", " cwqd * nvjh", " 2", " nvqn * dvjw", " pwgh - pfmr", " thbz + pzbs", " 2", " qnzw / qrlp", " 19", " sclc * zwms", " fmsf + hzlf", " crvp + vqpg", " dwdz + pncq", " vwtf * vrfr", " qhbw - vprz", " cfdc * vmbf", " glmp * bzhl", " wqhz * wbvr", " 2", " cgtj * fzqs", " 2", " 2", " svqq * smmg", " crdp * bngr", " fzjr + vfgn", " hscb - lmjw", " gdvr / crtp", " dlrd * zwrp", " 2", " bfbj / cjvd", " fqwv + jvzj", " fqgp * cfsz", " gmpt * tbgc", " jwmn * czhf", " tjvw + vsch", " tpfl * mbds", " vlqc / gzzt", " gdlr * zgnd", " sqnv * fjnp", " rhlv * dcgw", " 7", " 7", " lhrw - fbzw", " pndq + cpds", " dgng * bqbd", " svtg * nnvm", " lntp + bjft"]
  # "47221333683462 too high"
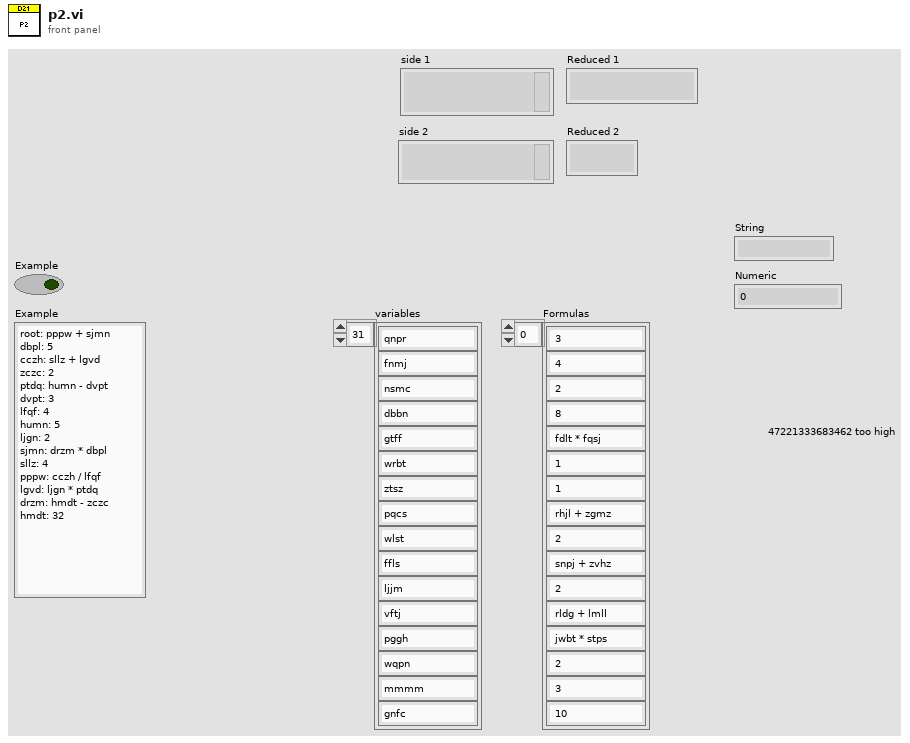
[diagram p1: front panel]
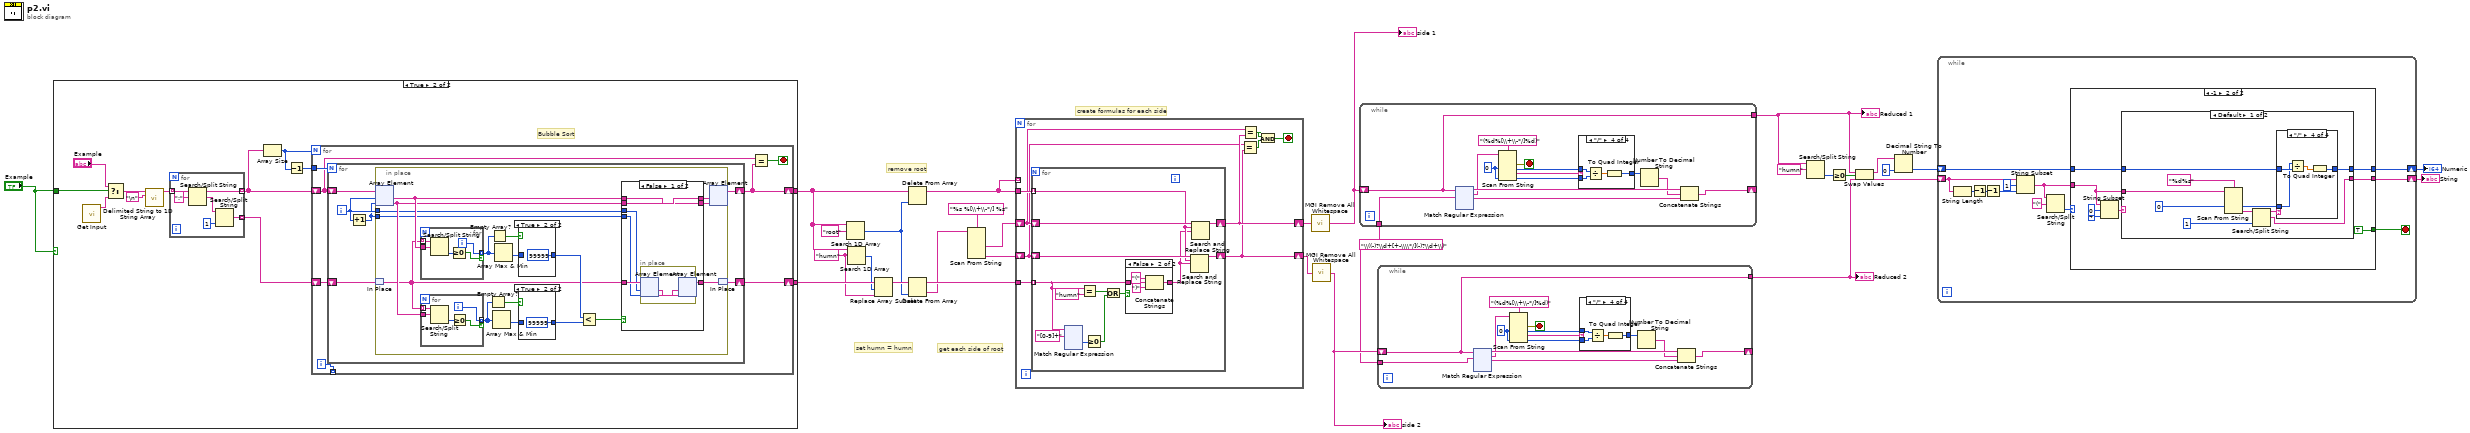
[diagram p0: block diagram]
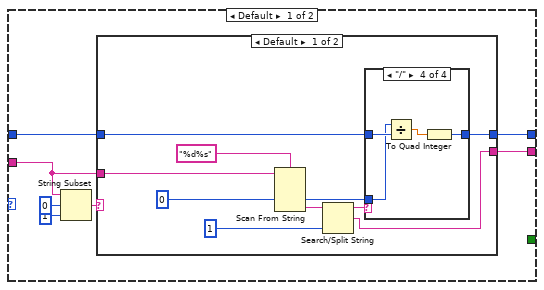
[diagram p2: hidden frame]
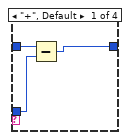
[diagram p3: hidden frame]
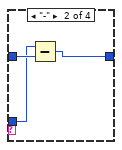
[diagram p4: hidden frame]
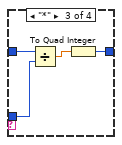
[diagram p5: hidden frame]
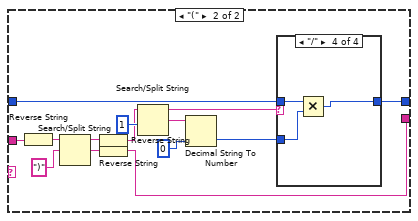
[diagram p6: hidden frame]
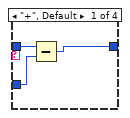
[diagram p7: hidden frame]
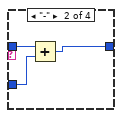
[diagram p8: hidden frame]
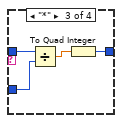
[diagram p9: hidden frame]
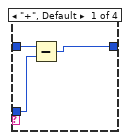
[diagram p10: hidden frame]
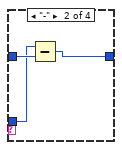
[diagram p11: hidden frame]
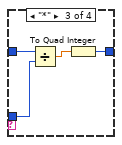
[diagram p12: hidden frame]
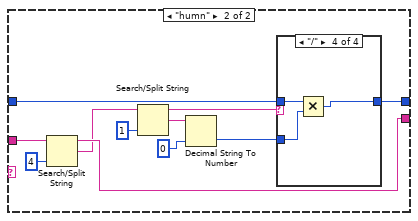
[diagram p13: hidden frame]
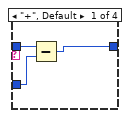
[diagram p14: hidden frame]
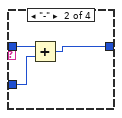
[diagram p15: hidden frame]
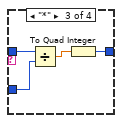
[diagram p16: hidden frame]
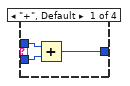
[diagram p17: hidden frame]
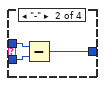
[diagram p18: hidden frame]
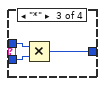
[diagram p19: hidden frame]
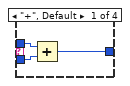
[diagram p20: hidden frame]
diagram:
  w12 = "\\((-)?\\d+[+-\\\\*/](-)?\\d+\\)" ("regular expression")
  w23 = "humn" ("element")
  # "get each side of root"
  # "remove root"
  # "create formulas for each side"
  # "set humn = humn"
  n1 = case shown="True" "Example" {
    tunnel: ["variables" w35] -> w22
    tunnel: ["Formulas" w34] -> w25
    tunnel: "Example" -> [_ w33]
    frame False {
    }
    frame True {
      # "Bubble Sort"
      n2 = call "Get Input.vi"() -> ("Input"=w44:string)  [unwired: 11 in]
      n3 = Select(t="Example", s=w33, f=w44) -> (s? t:f=w43:string)
      n4 = call <vilib>:"Delimited String to 1D String Array.vi"("delimiter"="\n", "delimited string"=w43) -> ("string array"=w40:string[])  [unwired: 9 in]
      n5 = for {
        tunnel: w40 -> [w105] mode=indexing
        tunnel: [w101] -> w37 mode=indexing
        tunnel: [w100] -> w36 mode=indexing
        n6 = Search/Split String(string=w105, search string/char (-)=":") -> (substring before match=w101:string, match + rest of string=w103:string)  [unwired: 1 in, 1 out]
        n7 = Search/Split String(string=w103, offset (0)=1) -> (match + rest of string=w100:string)  [unwired: 1 in, 2 out]
      }
      n8 = Array Size(array=w37) -> (size(s)=w38:i32)
      n9 = Decrement(x=w38) -> (x-1=w39:i32)
      n10 = for {
        N: w38 -> [_]
        tunnel: w39 -> [w50]
        shift-right: [w46] -> w35
        shift-left: w37 -> [w49]
        shift-right: [w47] -> w34
        shift-left: w36 -> [w48]
        tunnel: [w45] -> _ mode=indexing
        i -> [w45]
        stop <- w51 stop-if-true
        n11 = for {
          N: w50 -> [_]
          shift-right: [w52] -> w46
          shift-left: w49 -> [w57]
          shift-right: [w53] -> w47
          shift-left: w48 -> [w56]
          i -> [w55]
          n12 = Increment(x=w55) -> (x+1=w54:i32)
          n13 = in-place {
            in-place-border: w55 -> [w61]
            in-place-border: w54 -> [w60]
            n14 = in-place-array #1(w57, w55, w54) -> (w65:string, w64:string)
            n15 = in-place-match #2(w56) -> (w58:string[])
            n16 = for {
              tunnel: [w97] -> w73 mode=indexing if=w98
              tunnel: w65 -> [w96]
              tunnel: w58 -> [w95] mode=indexing
              i -> [w97]
              n17 = Search/Split String(string=w95, search string/char (-)=w96) -> (offset of match=w99:i32)  [unwired: 1 in, 2 out]
              n18 = Greater Or Equal To 0?(x=w99) -> (x >= 0?=w98:bool)
            }
            n19 = for {
              tunnel: [w90] -> w70 mode=indexing if=w91
              tunnel: w64 -> [w89]
              tunnel: w58 -> [w88] mode=indexing
              i -> [w90]
              n20 = Search/Split String(string=w88, search string/char (-)=w89) -> (offset of match=w92:i32)  [unwired: 1 in, 2 out]
              n21 = Greater Or Equal To 0?(x=w92) -> (x >= 0?=w91:bool)
            }
            n22 = Empty Array?(array=w70) -> (empty?=w71:bool)
            n23 = Empty Array?(array=w73) -> (empty?=w74:bool)
            n24 = Array Max & Min(array=w70) -> (min value=w68:i32)  [unwired: 3 out]
            n25 = Array Max & Min(array=w73) -> (min value=w72:i32)  [unwired: 3 out]
            n26 = case shown="True" w74 {
              tunnel: [w93 99999 ("min value")] -> w67
              tunnel: w72 -> [w93 _]
              frame False {
              }
              frame True {
              }
            }
            n27 = case shown="True" w71 {
              tunnel: [w86 99999 ("min value")] -> w69
              tunnel: w68 -> [w86 _]
              frame False {
              }
              frame True {
              }
            }
            n28 = Less?(x=w67, y=w69) -> (x < y?=w66:bool)
            n29 = case shown="False" w66 {
              tunnel: w65 -> [w79 w85]
              tunnel: w64 -> [w80 w84]
              tunnel: [w80 w85] -> w63
              tunnel: [w79 w84] -> w62
              tunnel: w58 -> [w78 w83]
              tunnel: w61 -> [w77 _]
              tunnel: w60 -> [w76 _]
              tunnel: [w75 w83] -> w59
              frame False {
                n30 = in-place {
                  n31 = in-place-array #3(w78, w77, w76) -> (w82:string, w81:string)
                  n32 = in-place-array #3(w81, w82) -> (w75:string[])  [unwired: 2 out]
                }
              }
              frame True {
              }
            }
            n33 = in-place-array #1(w63, w62) -> (w52:string[])  [unwired: 2 out]
            n34 = in-place-match #2(w59) -> (w53:string[])
          }
        }
        n35 = Equal?(x=w49, y=w46) -> (x = y?=w51:bool)
      }
    }
  }
  n36 = Search 1D Array(1D array=w22, element="root") -> (index of element=w17:i32)  [unwired: 1 in]
  n37 = Search 1D Array(1D array=w22, element=w23) -> (index of element=w24:i32)  [unwired: 1 in]
  n38 = Replace Array Subset(array=w25, new element=w23, index=w24) -> (w20:string[])
  n39 = Delete From Array(array=w22, index=w17) -> (array with subset deleted=w21:string[])  [unwired: 1 in, 1 out]
  n40 = Delete From Array(array=w20, index=w17) -> (deleted portion=w18:string, array with subset deleted=w19:string[])  [unwired: 1 in]
  n41 = Scan From String(format string="%s %[\\+\\-*/] %s", input string=w18) -> (output 1=w27:string, output 3=w26:string)  [unwired: 6 in, 3 out]
  n42 = for {
    tunnel: w19 -> [w114]
    tunnel: w21 -> [w113]
    shift-right: [w111] -> w16
    shift-left: w27 -> [w112]
    shift-right: [w110] -> w14
    shift-left: w26 -> [w109]
    tunnel: w21 -> [_] mode=indexing
    stop <- w106 stop-if-true
    n43 = for {
      tunnel: w114 -> [w120] mode=indexing
      tunnel: w113 -> [w125] mode=indexing
      shift-right: [w124] -> w111
      shift-left: w112 -> [w127]
      shift-right: [w123] -> w110
      shift-left: w109 -> [w126]
      n44 = xnode "Match Regular Expression"("input string"=w120, "regular expression"="[0-9]+") -> ("offset past match"=w116:i32)  [unwired: 4 in, 4 out]
      n45 = Equal?(x=w120, y="humn") -> (x = y?=w118:bool)
      n46 = Greater Or Equal To 0?(x=w116) -> (x >= 0?=w115:bool)
      n47 = Or(x=w118, y=w115) -> (x .or. y?=w117:bool)
      n48 = case shown="False" w117 {
        tunnel: [w245 w249] -> w122
        tunnel: w120 -> [w245 w248]
        frame True {
        }
        frame False {
          n49 = Concatenate Strings("(" ("string"), w248, ")" ("string")) -> (w249:string)
        }
      }
      n50 = Search and Replace String(input string=w126, search string=w125, replace string=w122) -> (result string=w123:string)  [unwired: 5 in, 3 out]
      n51 = Search and Replace String(input string=w127, search string=w125, replace string=w122) -> (result string=w124:string)  [unwired: 5 in, 3 out]
    }
    n52 = Equal?(x=w109, y=w110) -> (x = y?=w107:bool)
    n53 = Equal?(x=w112, y=w111) -> (x = y?=w108:bool)
    n54 = And(x=w108, y=w107) -> (x .and. y?=w106:bool)
  }
  n55 = call <userlib>:"MGI Remove All Whitespace.vi"("String"=w16) -> ("Trimmed String"=w15:string)
  "side 1" <- w15
  n56 = call <userlib>:"MGI Remove All Whitespace.vi"("String"=w14) -> ("Trimmed String"=w13:string)
  "side 2" <- w13
  n57 = while {
    shift-right: [w262] -> _
    shift-left: w15 -> [w253]
    tunnel: [w253] -> w8
    tunnel: w12 -> [w251]
    stop <- w254 stop-if-true
    w250 = i64 0
    n58 = xnode "Match Regular Expression"("input string"=w253, "regular expression"=w251) -> ("before match"=w263:string, "whole match"=w259:string, "after match"=w261:string)  [unwired: 4 in, 2 out]
    n59 = Scan From String(format string="(%d%[\\+\\-*/]%d)", input string=w259, default 1=w250, default 3=w250) -> (error out=w254:errorcluster, output 1=w252:i64, output 2=w258:string, output 3=w257:i64)  [unwired: 3 in, 2 out]
    n60 = case shown="\"/\"" w258 {
      tunnel: w252 -> [w265 w268 w271 w275]
      tunnel: w257 -> [w266 w269 w272 w276]
      tunnel: [w264 w267 w270 w273] -> w256
      frame "+", Default {
        n61 = Add(x=w265, y=w266) -> (x+y=w264:i64)
      }
      frame "-" {
        n62 = Subtract(x=w268, y=w269) -> (x-y=w267:i64)
      }
      frame "*" {
        n63 = Multiply(x=w271, y=w272) -> (x*y=w270:i64)
      }
      frame "/" {
        n64 = Divide(x=w275, y=w276) -> (x/y=w274:dbl)
        n65 = To Quad Integer(1:w274) -> (0:w273:i64)
      }
    }
    n66 = Number To Decimal String(number=w256) -> (decimal integer string=w255:string)  [unwired: 1 in]
    n67 = Concatenate Strings(w263, w255, w261) -> (w262:string)
  }
  "Reduced 1" <- w8
  n68 = while {
    shift-right: [w406] -> _
    shift-left: w13 -> [w397]
    tunnel: [w397] -> w7
    tunnel: w12 -> [w395]
    stop <- w398 stop-if-true
    w394 = i64 0 ("default value 1")
    n69 = xnode "Match Regular Expression"("input string"=w397, "regular expression"=w395) -> ("before match"=w407:string, "whole match"=w403:string, "after match"=w405:string)  [unwired: 4 in, 2 out]
    n70 = Scan From String(format string="(%d%[\\+\\-*/]%d)", input string=w403, default 1=w394, default 3=w394) -> (error out=w398:errorcluster, output 1=w396:i64, output 2=w402:string, output 3=w401:i64)  [unwired: 3 in, 2 out]
    n71 = case shown="\"/\"" w402 {
      tunnel: w396 -> [w409 w412 w415 w419]
      tunnel: w401 -> [w410 w413 w416 w420]
      tunnel: [w408 w411 w414 w417] -> w400
      frame "+", Default {
        n72 = Add(x=w409, y=w410) -> (x+y=w408:i64)
      }
      frame "-" {
        n73 = Subtract(x=w412, y=w413) -> (x-y=w411:i64)
      }
      frame "*" {
        n74 = Multiply(x=w415, y=w416) -> (x*y=w414:i64)
      }
      frame "/" {
        n75 = Divide(x=w419, y=w420) -> (x/y=w418:dbl)
        n76 = To Quad Integer(1:w418) -> (0:w417:i64)
      }
    }
    n77 = Number To Decimal String(number=w400) -> (decimal integer string=w399:string)  [unwired: 1 in]
    n78 = Concatenate Strings(w407, w399, w405) -> (w406:string)
  }
  "Reduced 2" <- w7
  n79 = Search/Split String(string=w8, search string/char (-)="humn") -> (offset of match=w10:i32)  [unwired: 1 in, 2 out]
  n80 = Greater Or Equal To 0?(x=w10) -> (x >= 0?=w9:bool)
  n81 = Swap Values(12:w8, 13:w9, 14:w7) -> (1:w5:string, 3:w4:string)
  n82 = Decimal String To Number(string=w5, default (0L)=i64 0 ("default (0 I32)")) -> (number=w6:i64)  [unwired: 1 in, 1 out]
  n83 = while {
    shift-right: [w548] -> w2
    shift-left: w4 -> [w546]
    shift-right: [w547] -> w1
    shift-left: w6 -> [w549]
    stop <- w538 stop-if-true
    n84 = String Length(string=w546) -> (length=w544:i32)
    n85 = Decrement(x=w544) -> (x-1=w543:i32)
    n86 = Decrement(x=w543) -> (x-1=w542:i32)
    n87 = String Subset(string=w546, offset (0)=1, length (rest)=w542) -> (substring=w540:string)
    n88 = Search/Split String(string=w540, search string/char (-)="(") -> (offset of match=w539:i32)  [unwired: 1 in, 2 out]
    n89 = case shown="-1" w539 {
      tunnel: w549 -> [w556 w615]
      tunnel: [w555 w614] -> w548
      tunnel: [w554 w613] -> w547
      tunnel: w540 -> [w552 w611]
      tunnel: [_ TRUE] -> w538
      frame Default {
        n90 = String Subset(string=w552, offset (0)=0, length (rest)=1 ("length (rest)")) -> (substring=w551:string)
        n91 = case shown="Default" w551 {
          tunnel: w556 -> [w562 w594]
          tunnel: [w558 w584] -> w555
          tunnel: [w557 w593] -> w554
          tunnel: w552 -> [w566 w592]
          frame Default {
            n92 = Scan From String(format string="%d%s", input string=w566, default 1=i64 0 ("default value 1")) -> (output 1=w561:i64, output 2=w563:string)  [unwired: 3 in, 3 out]
            n93 = Search/Split String(string=w563, offset (0)=1) -> (substring before match=w560:string, match + rest of string=w558:string)  [unwired: 1 in, 1 out]
            n94 = case shown="\"/\"" w560 {
              tunnel: w562 -> [w569 w572 w575 w579]
              tunnel: w561 -> [w568 w571 w574 w578]
              tunnel: [w567 w570 w573 w577] -> w557
              frame "+", Default {
                n95 = Subtract(x=w569, y=w568) -> (x-y=w567:i64)
              }
              frame "-" {
                n96 = Subtract(x=w571, y=w572) -> (x-y=w570:i64)
              }
              frame "*" {
                n97 = Divide(x=w575, y=w574) -> (x/y=w576:dbl)
                n98 = To Quad Integer(1:w576) -> (0:w573:i64)
              }
              frame "/" {
                n99 = Divide(x=w578, y=w579) -> (x/y=w580:dbl)
                n100 = To Quad Integer(1:w580) -> (0:w577:i64)
              }
            }
          }
          frame "(" {
            n101 = Reverse String(1:w592) -> (0:w591:string)
            n102 = Search/Split String(string=w591, search string/char (-)=")") -> (substring before match=w589:string, match + rest of string=w588:string)  [unwired: 1 in, 1 out]
            n103 = Reverse String(1:w589) -> (0:w582:string)
            n104 = Reverse String(1:w588) -> (0:w584:string)
            n105 = Search/Split String(string=w582, offset (0)=1) -> (substring before match=w583:string, match + rest of string=w581:string)  [unwired: 1 in, 1 out]
            n106 = Decimal String To Number(string=w581, default (0L)=i64 0 ("default (0 I32)")) -> (number=w586:i64)  [unwired: 1 in, 1 out]
            n107 = case shown="\"/\"" w583 {
              tunnel: w594 -> [w597 w600 w603 w607]
              tunnel: w586 -> [w596 w599 w602 w606]
              tunnel: [w595 w598 w601 w605] -> w593
              frame "+", Default {
                n108 = Subtract(x=w597, y=w596) -> (x-y=w595:i64)
              }
              frame "-" {
                n109 = Add(x=w600, y=w599) -> (x+y=w598:i64)
              }
              frame "*" {
                n110 = Divide(x=w603, y=w602) -> (x/y=w604:dbl)
                n111 = To Quad Integer(1:w604) -> (0:w601:i64)
              }
              frame "/" {
                n112 = Multiply(x=w607, y=w606) -> (x*y=w605:i64)
              }
            }
          }
        }
      }
      frame -1 {
        n113 = String Subset(string=w611, offset (0)=0, length (rest)=4 ("length (rest)")) -> (substring=w610:string)
        n114 = case shown="Default" w610 {
          tunnel: w615 -> [w621 w650]
          tunnel: [w617 w641] -> w614
          tunnel: [w616 w649] -> w613
          tunnel: w611 -> [w625 w643]
          frame Default {
            n115 = Scan From String(format string="%d%s", input string=w625, default 1=i64 0 ("default value 1")) -> (output 1=w620:i64, output 2=w622:string)  [unwired: 3 in, 3 out]
            n116 = Search/Split String(string=w622, offset (0)=1) -> (substring before match=w619:string, match + rest of string=w617:string)  [unwired: 1 in, 1 out]
            n117 = case shown="\"/\"" w619 {
              tunnel: w621 -> [w628 w631 w634 w638]
              tunnel: w620 -> [w627 w630 w633 w637]
              tunnel: [w626 w629 w632 w636] -> w616
              frame "+", Default {
                n118 = Subtract(x=w628, y=w627) -> (x-y=w626:i64)
              }
              frame "-" {
                n119 = Subtract(x=w630, y=w631) -> (x-y=w629:i64)
              }
              frame "*" {
                n120 = Divide(x=w634, y=w633) -> (x/y=w635:dbl)
                n121 = To Quad Integer(1:w635) -> (0:w632:i64)
              }
              frame "/" {
                n122 = Divide(x=w637, y=w638) -> (x/y=w639:dbl)
                n123 = To Quad Integer(1:w639) -> (0:w636:i64)
              }
            }
          }
          frame "humn" {
            n124 = Search/Split String(string=w643, offset (0)=4) -> (substring before match=w641:string, match + rest of string=w640:string)  [unwired: 1 in, 1 out]
            n125 = Search/Split String(string=w640, offset (0)=1) -> (substring before match=w645:string, match + rest of string=w644:string)  [unwired: 1 in, 1 out]
            n126 = Decimal String To Number(string=w644, default (0L)=i64 0 ("default (0 I32)")) -> (number=w647:i64)  [unwired: 1 in, 1 out]
            n127 = case shown="\"/\"" w645 {
              tunnel: w650 -> [w653 w656 w659 w663]
              tunnel: w647 -> [w652 w655 w658 w662]
              tunnel: [w651 w654 w657 w661] -> w649
              frame "+", Default {
                n128 = Subtract(x=w653, y=w652) -> (x-y=w651:i64)
              }
              frame "-" {
                n129 = Add(x=w656, y=w655) -> (x+y=w654:i64)
              }
              frame "*" {
                n130 = Divide(x=w659, y=w658) -> (x/y=w660:dbl)
                n131 = To Quad Integer(1:w660) -> (0:w657:i64)
              }
              frame "/" {
                n132 = Multiply(x=w663, y=w662) -> (x*y=w661:i64)
              }
            }
          }
        }
      }
    }
  }
  "String" <- w2
  "Numeric" <- w1
